vi "HAGAR_ECD.vi"() -> ()   [LabVIEW 2017]
uses:
  <vilib>/FPGAPlugInAG/cRIO-9035/niLvFpga_Close_cRIO-9035.vi
  <vilib>/rvi/errors/niLvFpgaAdjustHostInterfaceError.vi
  <vilib>/Utility/error.llb/Error Cluster From Error Code.vi
  GVZeitenZyklen_ECD.vi
  gvbooleschRT_ECD.vi
  GVHorstSP_ECD.vi
  GVMethodenwechsel_ECD.vi
  GVaktuelleTDMS_ECD.vi
  GVChroms_ECD.vi
  GVMetavariablen_ECD.vi
  GVMWHorst_ECD.vi
  GVVentilposition_ECD.vi
  GVHK1Hz_ECD.vi
  GVZwangs_ECD.vi
  GVZwangsMPV_ECD.vi
  GVTrapsMachs_ECD.vi
  GVECDs_ECD.vi
  GVAIs_ECD.vi
  GVHeizenLH_ECD.vi
  GVProbenvol_ECD.vi
  GVZwischenspeicher.vi
  <vilib>/rvi/interface/nirviCloseFPGA/nirviCloseFPGA.xnode
  FPGA Bitfiles/HAGAR-V_FPGATargetECD_FPGA-ProgrammECD_LbBtUh8SPQY.lvbitx
  FPGA_ECD/FPGA-Programm_ECD.vi
  <vilib>/rvi/interface/nirviReadWriteControl/nirviReadWriteControl.xnode
  <vilib>/rvi/interface/nirviMethod/nirviMethod.xnode
  <vilib>/NI_Real-Time Target Support.lvlib
  <vilib>/rvi/errors/niLvFpgaMergeErrorWithErrorCode.vi
  <vilib>/FPGAPlugInAG/cRIO-9035/niLvFpga_WriteFifo_cRIO-9035.vi
  NiFpgaLv.dll
panel:
  in  "Zyklus":enum16{"Mod0", "Mod1", "Mod2A", "Mod2B"}(ring)=enum."Mod1"
  in  "am Ende benutzen":bool
  in  "Methode speichern":bool
  out "ZyklusNummernGesamt":i32[](array[numeric])
  in  "veränderte Methode benutzen":bool
  in  "Methode verändern":bool
  out "ZyklusNummern":i32[](array[numeric])
  out "Big Ben, Methodenzeit, Zykluszeit0, Zykluszeit1, Zykluszeit2A, Zykluszeit2B":i32[](array[numeric])
  in  "global stop RT":bool
  in  "Methode":i32(ring) items=["Bedingsmethode", "Startmethode", "Meßmodus", "Shut-up-Methode", "Test", "HAG2 1/2", "Startmethode", "HAG2 1/2 Aufwärmen", "LicorDruckProfil1", "LicorDruckProfil2", "LicorDruckProfil0", "LicorDruckProfil3", "Kalibration-Meßmodus", "Kalibration-Meßmodus-II", "Kalibration-MesmodusIII", "Kalibration-Messmodus-IV", "Kalibration-ECD", "", "Kalibration-ECD-Blank"]
  in  "Registerkarte":T1(tab)
  out "SHOK?":bool[](array[boolean])
  out "schnelle Heizungen":string[](array[string])
  out "schnelle Heizungen":dbl[](array[numeric])
  out "HorstOK?":bool[](array[boolean])
  out "AIs3OK?":bool[](array[boolean])
  out "AIs1OK?":bool[](array[boolean])
  out "AIs1":dbl[](array[numeric])
  out "AIs1":string[](array[string])
  out "AIs2":string[](array[string])
  out "AIs3":string[](array[string])
  out "AIs2":dbl[](array[numeric])
  out "AIs3":dbl[](array[numeric])
  out "Metavariablen":string[](array[string])
  out "MVWerte":dbl[](array[numeric])
  out "MWHorst":dbl[](array[numeric])
  out "HorstRegler":string[](array[string])
  out "AIs2OK?":bool[](array[boolean])
  out "Ventilposition":i32=1 min=1 max=6 step=1
  out "MVOK?":bool[](array[boolean])
  out "CPU Total (%)":dbl
  in  "MVFixwert":dbl[](array[numeric])
  in  "MVFix?":bool[](array[boolean])
  in  "LH-Gruppe":bool[](array[boolean])=[FALSE, FALSE, FALSE, FALSE, FALSE, FALSE, FALSE, FALSE, FALSE, FALSE, FALSE, FALSE]
  out "LangsameHeizungen":string[](array[string])
  out "Housekeeping1":cluster{dbl[], dbl[]}(graph)
  in  "Zeitachse1":i32(ring)=1 items=["Zykluszeit [s] Mod0", "Zykluszeit [s] Mod1", "Zykluszeit [s] Mod2A", "Zykluszeit [s] Mod2B"]
  in  "dargestellte Größe 1":i32(ring)=1 items=["T1-Spare1", "T1-Spare2", "T1-StirlingKühlkopf [°C]", "T1-PreCol1 [°C]", "T1-PreCol2 [°C]", "T1-MainCol1a [°C]", "T1-MainCol1b [°C]", "T1-MainCol2a [°C]", "T1-MainCol2b [°C]", "T1-BronkhorstUntena [°C]", "T1-BronkhorstUntenb [°C]", "T1-BronkhorstObena [°C]", "T1-BronkhorstObenb [°C]", "T1-2Pos1B [°C]", "T1-Spare9", "T1-2Pos1A [°C]", "T1-Spare10", "T1-TurboPump [°C]", "T1-StirlingPlatine [°C]", "T1-Spare5", "T1-Spare6", "T1-Spare7", "T1-Inlet [°C]", "F1-MFM-Spare", "F1-MFM0D [mL]", "P1-HeliumHP [bara]", "P1-HeliumLP [bara]", "P1-PumpVordruck [mbara]", "TurboSpeed", "I1-MS-AC [A]", "I1-Trap1 [A]", "I1-Trap2 [A]", "T2-ECD1a", "T2-ECD1b", "T2-ECD2a", "T2-ECD2b", "T2-Col1a", "T2-Col1b", "T2-Col2a", "T2-Col2b", "T2-Spare1", "T2-Spare2", "T2-Spare3", "T2-Spare4", "T2-Spare5", "T2-Spare6", "T2-Spare7", "F2-MFM2A", "F2-MFM2B", "F2-MFM2C", "P2-N2O_HP", "P2-N2O_LP", "P2-CO2_HP", "P2-CO2_LP", "AI-Spare1", "FL-MFM1000mL", "AI-Spare3", "AI-Spare4", "StirlingAlarm", "StirlingEmerg.", "AI-Spare7", "AI-Spare8", "AI-Spare9", "FL-MFM30mL", "T0-DC/DC5", "I0-24V_M0", "I0-48V_M1", "I0-24V_M1", "I0-28V_M2", "T0-Spare3", "T0-Spare2", "T0-Spare4", "T0-DC/DC7", "I0-20V_Laptop", "I0-28V_M1", "I0-24V_M2", "I0-12V_Licor", "T0-Spare1", "T0-Drier", "T0-Spare5", "F0-MFM0A [L]", "TL-Licor_a", "P0-Span-HP", "P0-spare1", "P0-Stickstoff-LP", "P0-Helium-LP", "P0-Cal-HP", "P0-P9Tavco[bar]", "F0-MFM0B [L]", "TL-Licor_b", "P0-Span-LP", "P0-spare2", "P0-Stickstoff-HP", "P0-Helium-HP", "P0-Cal-LP", "F0-MFM3", "Trap1 [°C]", "Trap2 [°C]", "PreCol1 [°C]", "PreCol2 [°C]", "MainCol1 [°C]", "MainCol2 [°C]", "PrC0 [bara]", "PrC0-Licor [bara]", "PrC1-Säule1 [bara]", "PrC1-Säule2 [bara]", "MFC1-Sample [ml/min]", "PrC1-BackFlush1 [bara]", "PrC1-BackFlush2 [bara]", "MFC1-Reaktant [l/min]", "MFC2A[ml/min]", "MFC2B[ml/min]", "MFC2C[ul/min]", "PrC2A[bara]", "MFC2D[ml/min]", "MFC2E[ml/min]", "PrC2B[bara]"]
  out "Housekeeping2":cluster{dbl[], dbl[]}(graph)
  in  "Zeitachse2":i32(ring)=1 items=["Zykluszeit [s] Mod0", "Zykluszeit [s] Mod1", "Zykluszeit [s] Mod2A", "Zykluszeit [s] Mod2B"]
  in  "dargestellte Größe 2":i32(ring)=1 items=["T1-Spare1", "T1-Spare2", "T1-StirlingKühlkopf [°C]", "T1-PreCol1 [°C]", "T1-PreCol2 [°C]", "T1-MainCol1a [°C]", "T1-MainCol1b [°C]", "T1-MainCol2a [°C]", "T1-MainCol2b [°C]", "T1-BronkhorstUntena [°C]", "T1-BronkhorstUntenb [°C]", "T1-BronkhorstObena [°C]", "T1-BronkhorstObenb [°C]", "T1-2Pos1B [°C]", "T1-Spare9", "T1-2Pos1A [°C]", "T1-Spare10", "T1-TurboPump [°C]", "T1-StirlingPlatine [°C]", "T1-Spare5", "T1-Spare6", "T1-Spare7", "T1-Inlet [°C]", "F1-MFM-Spare", "F1-MFM0D [mL]", "P1-HeliumHP [bara]", "P1-HeliumLP [bara]", "P1-PumpVordruck [mbara]", "TurboSpeed", "I1-MS-AC [A]", "I1-Trap1 [A]", "I1-Trap2 [A]", "T2-ECD1a", "T2-ECD1b", "T2-ECD2a", "T2-ECD2b", "T2-Col1a", "T2-Col1b", "T2-Col2a", "T2-Col2b", "T2-Spare1", "T2-Spare2", "T2-Spare3", "T2-Spare4", "T2-Spare5", "T2-Spare6", "T2-Spare7", "F2-MFM2A", "F2-MFM2B", "F2-MFM2C", "P2-N2O_HP", "P2-N2O_LP", "P2-CO2_HP", "P2-CO2_LP", "AI-Spare1", "FL-MFM1000mL", "AI-Spare3", "AI-Spare4", "StirlingAlarm", "StirlingEmerg.", "AI-Spare7", "AI-Spare8", "AI-Spare9", "FL-MFM30mL", "T0-DC/DC5", "I0-24V_M0", "I0-48V_M1", "I0-24V_M1", "I0-28V_M2", "T0-Spare3", "T0-Spare2", "T0-Spare4", "T0-DC/DC7", "I0-20V_Laptop", "I0-28V_M1", "I0-24V_M2", "I0-12V_Licor", "T0-Spare1", "T0-Drier", "T0-Spare5", "F0-MFM0A [L]", "TL-Licor_a", "P0-Span-HP", "P0-spare1", "P0-Stickstoff-LP", "P0-Helium-LP", "P0-Cal-HP", "P0-P9Tavco[bar]", "F0-MFM0B [L]", "TL-Licor_b", "P0-Span-LP", "P0-spare2", "P0-Stickstoff-HP", "P0-Helium-HP", "P0-Cal-LP", "F0-MFM3", "Trap1 [°C]", "Trap2 [°C]", "PreCol1 [°C]", "PreCol2 [°C]", "MainCol1 [°C]", "MainCol2 [°C]", "PrC0 [bara]", "PrC0-Licor [bara]", "PrC1-Säule1 [bara]", "PrC1-Säule2 [bara]", "MFC1-Sample [ml/min]", "PrC1-BackFlush1 [bara]", "PrC1-BackFlush2 [bara]", "MFC1-Reaktant [l/min]", "MFC2A[ml/min]", "MFC2B[ml/min]", "MFC2C[ul/min]", "PrC2A[bara]", "MFC2D[ml/min]", "MFC2E[ml/min]", "PrC2B[bara]"]
  out "Detektor 2":cluster{dbl[], dbl[]}[](graph)
  in  "Detektor":i32(ring) items=["ECD1", "ECD2"]
  in  "HK1YMin":dbl
  in  "HK1YMax":dbl=100.0
  in  "HK2YMin":dbl
  in  "HK2YMax":dbl=100.0
  in  "DetYMin":dbl
  in  "DetYMax":dbl=100.0
  in  "NeuerRefstrom":bool
  in  "RefStromECD1":i16=800 min=0 max=2500 step=1
  in  "RefStromECD2":i16=2100 min=0 max=2500 step=1
  out "schnelleAnzeige":cluster{dbl[], dbl[]}(graph)
  in  "TafelWischen!":bool
  in  "dargestellte Größe 3":i32(ring)=1 items=["Trap1 [°C]", "Trap2 [°C]", "PreCol1 [°C]", "PreCol2 [°C]", "MainCol1 [°C]", "MainCol2 [°C]", "PrC0 [bara]", "PrC0-Licor [bara]", "PrC1-Säule1 [bara]", "PrC1-Säule2 [bara]", "MFC1-Sample [ml/min]", "PrC1-BackFlush1 [bara]", "PrC1-BackFlush2 [bara]", "MFC1-Reaktant [l/min]", "MFC2A[ml/min]", "MFC2B[ml/min]", "MFC2C[ul/min]", "PrC2A[bara]", "MFC2D[ml/min]", "MFC2E[ml/min]", "PrC2B[bara]"]
  in  "An/Aus":bool
  out "TDMSwriteECD":errorcluster
  out "AIsFIFOread":errorcluster
  out "MWTrapsMachs":errorcluster
  out "TDMSwriteHK":errorcluster
  out "TDMScloseHK":errorcluster
  out "TDMSopenHK":errorcluster
  out "TDMScloseECD2":errorcluster
  out "TDMSopenECD2":errorcluster
  out "TDMScloseECD1":errorcluster
  out "TDMSopenECD1":errorcluster
  out "FIFOwriteRS485":errorcluster
  out "SerielleKomm.":errorcluster
  out "LH":errorcluster
  out "Zyklus":errorcluster
  out "ECD1dataBackup":errorcluster
  out "ECD2dataBackup":errorcluster
  # "Zyklen:   ===>>"
  # "MS"
  # "ECD1"
  # "ECD2"
  # "Zykluszeiten:   ===>>"
  # "MS"
  # "ECD1"
  # "ECD2"
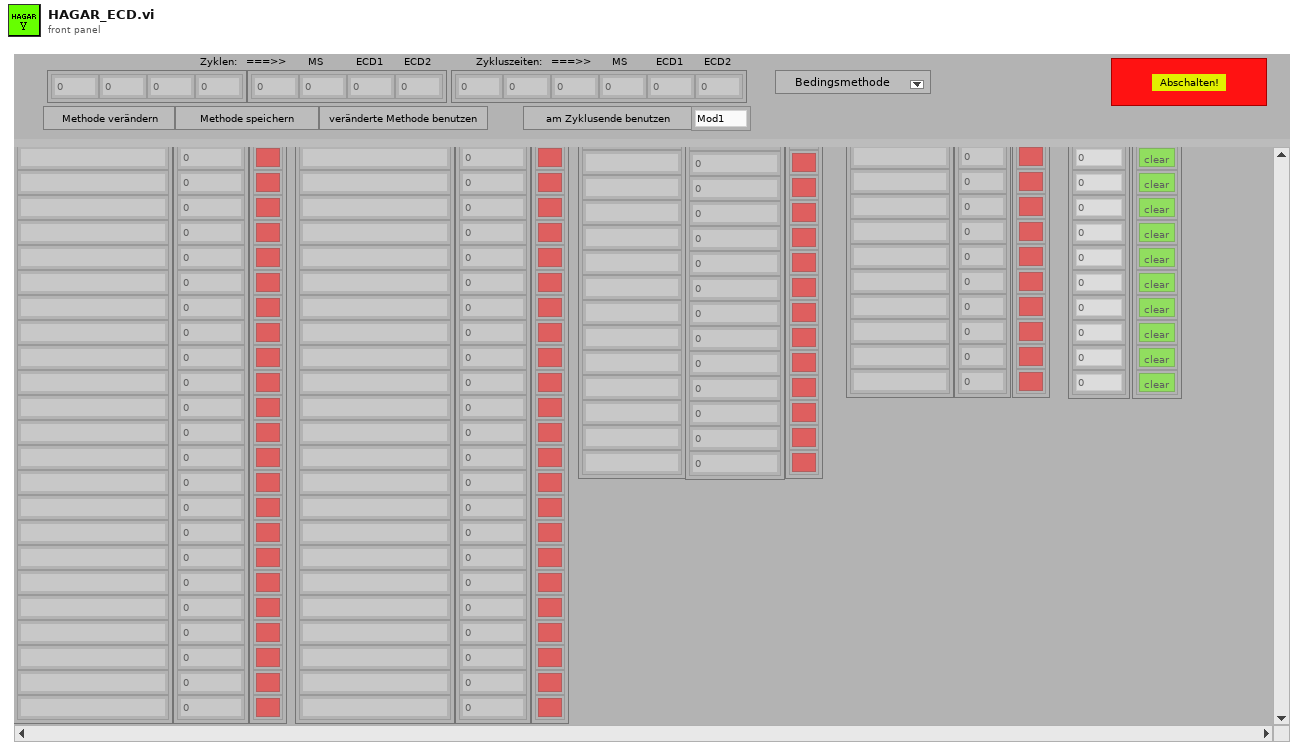
[diagram p1: front panel]
types:
  T1 = enum32{"Tabellen", "Heizungen gruppieren", "Bilder", "schnelle Bilder", "LICÖRchen", "Ups! Fehler"}
  T2 = cluster{"Zykluslängen [s]":dbl[], "ZeitpktDIOsMod0":dbl[], "ZeitpktDIOsMod1":dbl[], "ZeitpktDIOsMod2A":dbl[], "ZeitpktDIOsMod2B":dbl[], "DIOsSPMod0":bool[][], "DIOsSPMod1":bool[][], "DIOsSPMod2A":bool[][], "DIOsSPMod2B":bool[][], "Mod0HorstZeitpkt":dbl[], "Mod1HorstZeitpkt":dbl[], "Mod2AHorstZeitpkt":dbl[], "Mod2BHorstZeitpkt":dbl[], "HorstSPMod0":dbl[][], "HorstSPMod1":dbl[][], "HorstSPMod2A":dbl[][], "HorstSPMod2B":dbl[][], "LHSetpoints":dbl[], "LHHeizen?":bool[], "ZPktFPGABoolesch":dbl[], "FPGABoolesch":bool[][], "ZeitpktFPGAPID":dbl[], "FPGAPID":cluster{"d0":fxp<+/-,18,18>, "d1":fxp<+/-,21,21>}[][], "ZeitpktFPGAFixp":dbl[], dbl[][], "t_PreMach1":dbl[], "T_PreMach1":dbl[], "t_PreMach2":dbl[], "T_PreMach2":dbl[], "PIDs für \"träge\" Heizungen":cluster{"proportional gain (Kc)":dbl, "integral time (Ti, min)":dbl, "derivative time (Td, min)":dbl}[], "Zwangsbedingungen":dbl[][], "Dateien fürs MS schicken?":bool, "ZeitpunkteMPV":dbl[], "SPMPV":i32[], "ZeitpktMS-1":dbl, "ZeitpktMS-2":dbl, "Int.Start1":dbl, "Int.Stop1":dbl, "Int.Start2":dbl, "Int.Stop2":dbl, "Methodenname":string, "t_MainMach1":dbl[], "T_MainMach1":dbl[], "t_MainMach2":dbl[], "T_MainMach2":dbl[]}[]
  T3 = cluster{"DIOsMod0Nr":i32[], "DIOsMod1Nr":i32[], "DIOsMod2ANr":i32[], "DIOsMod2BNr":i32[], "AIsLH":i32[], "AnzahlRegler/Modul":i32[], "Regler für den Probenfluß":i32, "SPvorgebenMod0":string[], "SPvorgebenMod1":string[], "SPvorgebenMod2A":string[], "SPvorgebenMod2B":string[], "MWAntwortMod0":string[], "MWAntwortMod1":string[], "MWAntwortMod2A":string[], "MWAntwortMod2B":string[], "FaktorMod0":dbl[], "FaktorMod1":dbl[], "FaktorMod2A":dbl[], "FaktorMod2B":dbl[], "MWabfragenMod0":string[], "MWabfragenMod1":string[], "MWabfragenMod2A":string[], "MWabfragenMod2B":string[], "Modul1/AI koeff":dbl[][], "Modul2/AI koeff":dbl[][], "Modul3/AI koeff":dbl[][], "Traps/MachsKoeff T(R)":dbl[][], "Modul1/AIsNamen":string[], "Modul2/AIsNamen":string[], "Modul3/AIsNamen":string[], "DIOsMod0Name":string[], "DIOsMod1Name":string[], "DIOsMod2AName":string[], "DIOsMod2BName":string[], "ReglerNameMod0":string[], "ReglerNameMod1":string[], "ReglerNameMod2A":string[], "ReglerNameMod2B":string[], "Startmethode":i32, "Dateiordner Housekeeping":path, "Dateiname Housekeeping":string, "DateiordnerECD1":path, "DateinameECD1":string, "DateiordnerECD2":path, "DateinameECD2":string, "LangsameHeizungen":string[], "ModuleLH":i32[], "Metavariablen":string[], "Modul1/AI sicherer Bereich":dbl[][], "Modul2/AI sicherer Bereich":dbl[][], "Modul3/AI sicherer Bereich":dbl[][], "Traps/Machs sicherer Bereich":dbl[][], "ReglerMod0 sicherer Bereich":dbl[][], "ReglerMod1 sicherer Bereich":dbl[][], "ReglerMod2A sicherer Bereich":dbl[][], "ReglerMod2B sicherer Bereich":dbl[][], "Metavariablen grüner Bereich":dbl[][], "Traps/MachsKoeff R(U)":dbl[][], "LHGruppe":bool[]}
  T4 = enum16{"open", "replace", "create", "open or create", "replace or create", "replace or create with confirmation"}
  T5 = cluster{"Zyklus1":i32, "Zeitachse1":i32, "dargestellte Größe 1":i32, "Zyklus2":i32, "Zeitachse2":i32, "dargestellte Größe 2":i32}
  T6 = cluster{"DIOsMod0Name":string[], "DIOsMod1Name":string[], "DIOsMod2AName":string[], "DIOsMod2BName":string[], "ReglerNameMod0":string[], "ReglerNameMod1":string[], "ReglerNameMod2A":string[], "ReglerNameMod2B":string[], "LangsameHeizungen":string[]}
  T7 = cluster{"Zykluslängen [s]":dbl[], "ZeitpktDIOsMod0":dbl[], "ZeitpktDIOsMod1":dbl[], "ZeitpktDIOsMod2A":dbl[], "ZeitpktDIOsMod2B":dbl[], "DIOsSPMod0":bool[][], "DIOsSPMod1":bool[][], "DIOsSPMod2A":bool[][], "DIOsSPMod2B":bool[][], "Mod0HorstZeitpkt":dbl[], "Mod1HorstZeitpkt":dbl[], "Mod2AHorstZeitpkt":dbl[], "Mod2BHorstZeitpkt":dbl[], "HorstSPMod0":dbl[][], "HorstSPMod1":dbl[][], "HorstSPMod2A":dbl[][], "HorstSPMod2B":dbl[][], "LHSetpoints":dbl[], "LHHeizen?":bool[], "ZPktFPGABoolesch":dbl[], "FPGABoolesch":bool[][], "ZeitpktFPGAPID":dbl[], "FPGAPID":cluster{"d0":fxp<+/-,18,18>, "d1":fxp<+/-,21,21>}[][], "ZeitpktFPGAFixp":dbl[], dbl[][], "t_PreMach1":dbl[], "T_PreMach1":dbl[], "t_PreMach2":dbl[], "T_PreMach2":dbl[], "PIDs für \"träge\" Heizungen":cluster{"proportional gain (Kc)":dbl, "integral time (Ti, min)":dbl, "derivative time (Td, min)":dbl}[], "Zwangsbedingungen":dbl[][], "Dateien fürs MS schicken?":bool, "ZeitpunkteMPV":dbl[], "SPMPV":i32[], "ZeitpktMS-1":dbl, "ZeitpktMS-2":dbl, "Int.Start1":dbl, "Int.Stop1":dbl, "Int.Start2":dbl, "Int.Stop2":dbl, "Methodenname":string, "t_MainMach1":dbl[], "T_MainMach1":dbl[], "t_MainMach2":dbl[], "T_MainMach2":dbl[]}
  T8 = cluster{"Modul1/AI sicherer Bereich":dbl[][], "Modul2/AI sicherer Bereich":dbl[][], "Modul3/AI sicherer Bereich":dbl[][], "Traps/Machs sicherer Bereich":dbl[][], dbl[][], "Metavariablen grüner Bereich":dbl[][]}
  T9 = cluster{"created path":path, "created path":path}
  T10 = cluster{"created path":path, "created path":path, "created path":path, "Dateiname Housekeeping":string, "DateinameECD1":string, "DateinameECD2":string, "tdms0":refnum<k34>, "tdms1":refnum<k34>, "tdms0":refnum<k34>, "tdms1":refnum<k34>, "tdms0":refnum<k34>, "tdms1":refnum<k34>}
  T11 = cluster{"d0":fxp<+/-,18,18>, "d1":fxp<+/-,21,21>}[][]
  T12 = cluster{"proportional gain (Kc)":dbl, "integral time (Ti, min)":dbl, "derivative time (Td, min)":dbl}[]
  T13 = cluster{cluster{"ZeitpktDIOsMod2B":dbl[]}[], cluster{"DIOsSPMod2B":bool[][]}[], cluster{"Mod2BHorstZeitpkt":dbl[]}[], cluster{"HorstSPMod2B":dbl[][]}[], "LHHeizen?":bool[], "ZPktFPGABoolesch":dbl[], "FPGABoolesch":bool[][], "ZeitpktFPGAPID":dbl[], "FPGAPID":cluster{"d0":fxp<+/-,18,18>, "d1":fxp<+/-,21,21>}[][], "ZeitpktFPGAFixp":dbl[], dbl[][], "t_PreMach1":dbl[], "T_PreMach1":dbl[], "t_PreMach2":dbl[], "T_PreMach2":dbl[], "ZeitpunkteMPV":dbl[], "SPMPV":i32[], "t_MainMach1":dbl[], "T_MainMach1":dbl[], "t_MainMach2":dbl[], "T_MainMach2":dbl[]}
  T14 = cluster{"Zykluslängen [s]":dbl[], "ZeitpktDIOsMod0":dbl[], "ZeitpktDIOsMod1":dbl[], "ZeitpktDIOsMod2A":dbl[], "ZeitpktDIOsMod2B":dbl[], "DIOsSPMod0":bool[][], "DIOsSPMod1":bool[][], "DIOsSPMod2A":bool[][], "DIOsSPMod2B":bool[][], "Mod0HorstZeitpkt":dbl[], "Mod1HorstZeitpkt":dbl[], "Mod2AHorstZeitpkt":dbl[], "Mod2BHorstZeitpkt":dbl[], "HorstSPMod0":dbl[][], "HorstSPMod1":dbl[][], "HorstSPMod2A":dbl[][], "HorstSPMod2B":dbl[][], "LangsameHeizungenSP":dbl[], "LHHeizen?":bool[], "ZPktFPGABoolesch":dbl[], "FPGABoolesch":bool[][], "ZeitpktFPGAPID":dbl[], "FPGAPID":cluster{"d0":fxp<+/-,18,18>, "d1":fxp<+/-,21,21>}[][], "ZeitpktFPGAFixp":dbl[], "FPGAFixp":dbl[][], "t_PreMach1":dbl[], "T_PreMach1":dbl[], "t_PreMach2":dbl[], "T_PreMach2":dbl[], "PIDs für \"träge\" Heizungen":cluster{"proportional gain (Kc)":dbl, "integral time (Ti, min)":dbl, "derivative time (Td, min)":dbl}[], "Zwangsbedingungen":dbl[][], "MS-Daten?":bool, "ZeitpunkteMPV":dbl[], "SetpointMPV":i32[], "ZeitpktMS-1":dbl, "ZeitpktMS-2":dbl, "Int.Start1":dbl, "Int.Stop1":dbl, "Int.Start2":dbl, "Int.Stop2":dbl, "Methodenname":string, "t_MainMach1":dbl[], "T_MainMach1":dbl[], "t_MainMach2":dbl[], "T_MainMach2":dbl[]}
  T15 = cluster{"ZyklusNummern":i32[], "ZeilennummernDIOs":i32[], "ZwangsDIO?":cluster{bool[]}[], "ZeilennummernHorst":i32[], "ZwangsHorst?":cluster{bool[]}[], "ZeileFPGABoolesch":i32, "ZwangsFPGABoolesch?":bool[], "ZeileFPGAPID":i32, "ZeileFPGAFixp":i32, "ZeilePreMach1":i32, "ZeilePreMach2":i32, "ZeilennummerMPV":i32, "ZeileMainMach1":i32, "ZeileMainMach2":i32, "ZwangsMPV?":bool}
  T16 = typedef "NI_Real-Time Target Support.lvlib/RT CPU Load.ctl" = cluster{"Total (%)":dbl, "Time Critical (%)":dbl, "Timed Structures (%)":dbl, "High (%)":dbl, "Above Normal (%)":dbl, "Normal (%)":dbl, "Background (%)":dbl, "Idle (%)":dbl, "ISR (%)":dbl}
  T17 = cluster{"ZyklusNummern":i32[], i32[], "ZwangsDIO?":cluster{bool[]}[], i32[], "ZwangsHorst?":cluster{bool[]}[], i32, "ZwangsFPGABoolesch?":bool[], i32, i32, "ZeileMach":i32, "ZeileMach":i32, i32, "ZeileMach":i32, "ZeileMach":i32, "ZwangsMPV?":bool}
  T18 = cluster{string[], string[], string[], dbl[], dbl[], dbl[]}
  T19 = cluster{"Befehle1":string[], "Befehle2":string[], "Befehle3":string[]}
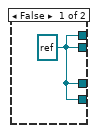
[diagram p2: hidden frame]
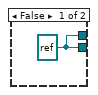
[diagram p3: hidden frame]
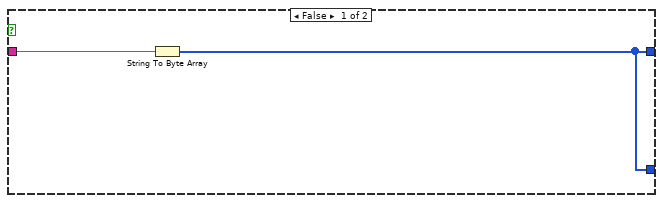
[diagram p6: hidden frame]
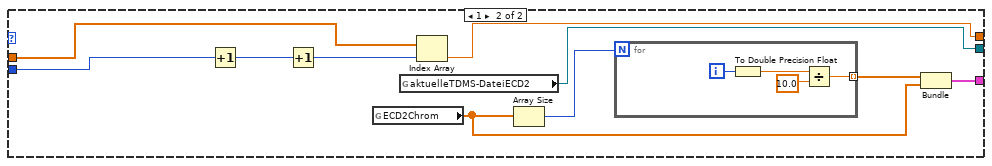
[diagram p16: hidden frame]
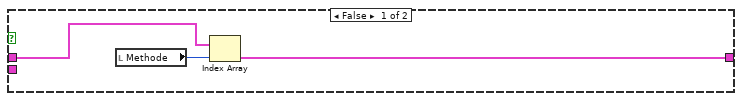
[diagram p17: hidden frame]
diagram:
  w2 = path "c:/methoden.pery" ("Datei (Dialog verwenden)")
  w3 = path "c:/einstellungen.pery" ("Datei (Dialog verwenden)")
  n1 = Open/Create/Replace File(file path (use dialog)=w3, operation (0:open)=T4."open" ("Operation (0:Öffnen)")) -> (refnum out=w15:refnum<file>)  [unwired: 4 in, 2 out]
  n2 = Open/Create/Replace File(file path (use dialog)=w2, operation (0:open)=T4."open" ("Operation (0:Öffnen)")) -> (refnum out=w11:refnum<file>)  [unwired: 4 in, 2 out]
  n3 = Read from Binary File(5:T3 {"DIOsMod0Nr"=[], "DIOsMod1Nr"=[], "DIOsMod2ANr"=[], "DIOsMod2BNr"=[], "AIsLH"=[], "AnzahlRegler/Modul"=[], "Regler für den Probenfluß"=0, "SPvorgebenMod0"=[], "SPvorgebenMod1"=[], "SPvorgebenMod2A"=[], "SPvorgebenMod2B"=[], "MWAntwortMod0"=[], "MWAntwortMod1"=[], "MWAntwortMod2A"=[], "MWAntwortMod2B"=[], "FaktorMod0"=[], "FaktorMod1"=[], "FaktorMod2A"=[], "FaktorMod2B"=[], "MWabfragenMod0"=[], "MWabfragenMod1"=[], "MWabfragenMod2A"=[], "MWabfragenMod2B"=[], "Modul1/AI koeff"=[], "Modul2/AI koeff"=[], "Modul3/AI koeff"=[], "Traps/MachsKoeff T(R)"=[], "Modul1/AIsNamen"=[], "Modul2/AIsNamen"=[], "Modul3/AIsNamen"=[], "DIOsMod0Name"=[], "DIOsMod1Name"=[], "DIOsMod2AName"=[], "DIOsMod2BName"=[], "ReglerNameMod0"=[], "ReglerNameMod1"=[], "ReglerNameMod2A"=[], "ReglerNameMod2B"=[], "Startmethode"=0, "Dateiordner Housekeeping"=path "", "Dateiname Housekeeping"="", "DateiordnerECD1"=path "", "DateinameECD1"="", "DateiordnerECD2"=path "", "DateinameECD2"="", "LangsameHeizungen"=[], "ModuleLH"=[], "Metavariablen"=[], "Modul1/AI sicherer Bereich"=[], "Modul2/AI sicherer Bereich"=[], "Modul3/AI sicherer Bereich"=[], "Traps/Machs sicherer Bereich"=[], "ReglerMod0 sicherer Bereich"=[], "ReglerMod1 sicherer Bereich"=[], "ReglerMod2A sicherer Bereich"=[], "ReglerMod2B sicherer Bereich"=[], "Metavariablen grüner Bereich"=[], "Traps/MachsKoeff R(U)"=[], "LHGruppe"=[]} ("output cluster"), 11:w15) -> (2:w13:T3, 3:w14:refnum<file>)  [unwired: 4 in, 2 out]
  n4 = Read from Binary File(5:T2 [], 11:w11) -> (2:w9:T2, 3:w10:refnum<file>)  [unwired: 4 in, 2 out]
  n5 = Close File(refnum=w14) -> ()  [unwired: 1 in, 2 out]
  n6 = Close File(refnum=w10) -> ()  [unwired: 1 in, 2 out]
  n7 = flat-sequence {
    tunnel: [w86] -> w42
    tunnel: [w146] -> w41
    tunnel: [w89] -> w39
    tunnel: [w279] -> w38
    tunnel: [w281] -> w37
    tunnel: [w273] -> w36
    tunnel: [w280] -> w35
    tunnel: [w203] -> w34
    tunnel: [w272] -> w33
    tunnel: [w271] -> w32
    tunnel: [w265] -> w31
    tunnel: [w206] -> w30
    tunnel: [w180] -> w29
    tunnel: [w278] -> w28
    tunnel: [w270] -> w27
    tunnel: [w269] -> w26
    tunnel: [w261] -> w25
    tunnel: [w260] -> w24
    tunnel: [w259] -> w23
    tunnel: [w258] -> w22
    tunnel: [w257] -> w21
    tunnel: [w256] -> w20
    tunnel: [w253] -> w19
    tunnel: [w235] -> w18
    tunnel: w13 -> [w128]
    tunnel: [w234] -> w17
    tunnel: w9 -> [w147]
    tunnel: [w146] -> w8
    tunnel: [w128] -> w7
    tunnel: [w97] -> w6
    tunnel: w3 -> [w83]
    tunnel: w2 -> [w79]
    tunnel: [w60] -> w1
    tunnel: w42 -> [w347]
    tunnel: w41 -> [w420]
    tunnel: [w347] -> w40
    tunnel: w39 -> [_]
    tunnel: w38 -> [w378]
    tunnel: w37 -> [w377]
    tunnel: w36 -> [w379]
    tunnel: w35 -> [w376]
    tunnel: w34 -> [w351]
    tunnel: w33 -> [w346]
    tunnel: w32 -> [w343]
    tunnel: w31 -> [w340]
    tunnel: w30 -> [w341]
    tunnel: w29 -> [w344]
    tunnel: w28 -> [w418]
    tunnel: w27 -> [w349]
    tunnel: w26 -> [w419]
    tunnel: w25 -> [w322]
    tunnel: w24 -> [w321]
    tunnel: w23 -> [w320]
    tunnel: w22 -> [w416]
    tunnel: w21 -> [w415]
    tunnel: w20 -> [w414]
    tunnel: w19 -> [w368]
    tunnel: w18 -> [w350]
    tunnel: w17 -> [w339]
    tunnel: w9 -> [w338]
    tunnel: w8 -> [w336]
    tunnel: w7 -> [_]
    tunnel: w6 -> [w315]
    tunnel: w1 -> [w314]
    tunnel: w40 -> [w1212]
    frame #0 {
      w43 = string[] ["x", "x", "x", "x"] ("write")
      w56 = "config" ("string")
      w78 = string[] ["Trap1 [°C]", "Trap2 [°C]", "PreCol1 [°C]", "PreCol2 [°C]", "MainCol1 [°C]", "MainCol2 [°C]"]
      w148 = TRUE
      w162 = 0.0 ("Probenvol.1")
      w169 = dbl[] [-1.0] ("ECD1MW")
      w170 = FALSE ("ECD1Empfangen?")
      w276 = string[] ["Big Ben [s]", "Methodenzeit [s]", "Zykluszeit [s] Mod0", "Zykluszeit [s] Mod1", "Zykluszeit [s] Mod2A", "Zykluszeit [s] Mod2B"]
      w266 = FALSE ("Undefinierte Werte möglich")
      w267 = FALSE ("global stop RT")
      n8 = for {
        tunnel: [w309] -> w274 mode=indexing
        tunnel: w147 -> [w310] mode=indexing
        n9 = Unbundle(w310) -> ("Methodenname"=w309:string)  [unwired: 44 out]
      }
      n10 = Unbundle(w128) -> ("DIOsMod0Nr"=w190:i32[], "DIOsMod1Nr"=w189:i32[], "DIOsMod2ANr"=w188:i32[], "DIOsMod2BNr"=w187:i32[], "AIsLH"=w177:i32[], "AnzahlRegler/Modul"=w180:i32[], "Regler für den Probenfluß"=w234:i32, "SPvorgebenMod0"=w233:string[], "SPvorgebenMod1"=w232:string[], "SPvorgebenMod2A"=w231:string[], "SPvorgebenMod2B"=w230:string[], "MWAntwortMod0"=w229:string[], "MWAntwortMod1"=w228:string[], "MWAntwortMod2A"=w227:string[], "MWAntwortMod2B"=w226:string[], "FaktorMod0"=w225:dbl[], "FaktorMod1"=w224:dbl[], "FaktorMod2A"=w223:dbl[], "FaktorMod2B"=w222:dbl[], "MWabfragenMod0"=w221:string[], "MWabfragenMod1"=w220:string[], "MWabfragenMod2A"=w219:string[], "MWabfragenMod2B"=w218:string[], "Modul1/AI koeff"=w217:dbl[][], "Modul2/AI koeff"=w216:dbl[][], "Modul3/AI koeff"=w215:dbl[][], "Traps/MachsKoeff T(R)"=w214:dbl[][], "Modul1/AIsNamen"=w213:string[], "Modul2/AIsNamen"=w212:string[], "Modul3/AIsNamen"=w211:string[], "DIOsMod0Name"=w126:string[], "DIOsMod1Name"=w127:string[], "DIOsMod2AName"=w125:string[], "DIOsMod2BName"=w124:string[], "ReglerNameMod0"=w139:string[], "ReglerNameMod1"=w138:string[], "ReglerNameMod2A"=w137:string[], "ReglerNameMod2B"=w136:string[], "Startmethode"=w146:i32, "Dateiordner Housekeeping"=w65:path, "Dateiname Housekeeping"=w210:string, "DateiordnerECD1"=w70:path, "DateinameECD1"=w209:string, "DateiordnerECD2"=w62:path, "DateinameECD2"=w208:string, "LangsameHeizungen"=w207:string[], "ModuleLH"=w202:i32[], "Metavariablen"=w141:string[], "Modul1/AI sicherer Bereich"=w101:dbl[][], "Modul2/AI sicherer Bereich"=w100:dbl[][], "Modul3/AI sicherer Bereich"=w99:dbl[][], "Traps/Machs sicherer Bereich"=w98:dbl[][], "ReglerMod0 sicherer Bereich"=w96:dbl[][], "ReglerMod1 sicherer Bereich"=w95:dbl[][], "ReglerMod2A sicherer Bereich"=w94:dbl[][], "ReglerMod2B sicherer Bereich"=w93:dbl[][], "Metavariablen grüner Bereich"=w91:dbl[][], "LHGruppe"=w85:bool[])  [unwired: 1 out]
      "Metavariablen" <- w141
      "LangsameHeizungen" <- w207
      n11 = Initialize Array(0, 4 ("Dimension")) -> (w163:i32[])
      n12 = Initialize Array(0.0 ("Element"), 6 ("Dimension")) -> (w166:dbl[])
      n13 = global write "GVMethodenwechsel_ECD.vi" "Methodenwechsel?"(FALSE ("Methodenwechsel?")) -> ()
      n14 = local write "NeuerRefstrom"(FALSE ("NeuerRefstrom")) -> ()
      n15 = property on="dargestellte Größe 2" class="Ring (strikt)"("AllowUndefVals"=w266) -> ()  [unwired: 2 in, 2 out]
      n16 = property on="Zeitachse2" class="Ring (strikt)"("AllowUndefVals"=w266) -> ()  [unwired: 2 in, 2 out]
      n17 = property on="Zeitachse1" class="Ring (strikt)"("AllowUndefVals"=w266) -> ()  [unwired: 2 in, 2 out]
      n18 = property on="dargestellte Größe 1" class="Ring (strikt)"("AllowUndefVals"=w266) -> ()  [unwired: 2 in, 2 out]
      n19 = property on="Methode" class="Ring (strikt)"("AllowUndefVals"=w266) -> ()  [unwired: 2 in, 2 out]
      n20 = global write "GVProbenvol_ECD.vi" "Probenvol.1"(w162) -> ()
      n21 = global write "GVProbenvol_ECD.vi" "Probenvol.2"(w162) -> ()
      n22 = global write "GVECDs_ECD.vi" "ECD1MW"(w169) -> ()
      n23 = global write "GVECDs_ECD.vi" "ECD2MW"(w169) -> ()
      n24 = global write "GVECDs_ECD.vi" "ECD1Empfangen?"(w170) -> ()
      n25 = global write "GVECDs_ECD.vi" "ECD2Empfangen?"(w170) -> ()
      n26 = local write "global stop RT"(w267) -> ()
      n27 = global write "gvbooleschRT_ECD.vi" "global stop RT"(w267) -> ()
      n28 = global write "GVZeitenZyklen_ECD.vi" "ZyklusNummern"(w163) -> ()
      n29 = global write "GVZeitenZyklen_ECD.vi" "ZyklusNummernGesamt"(w163) -> ()
      n30 = global write "GVZeitenZyklen_ECD.vi" "Big Ben, Methodenzeit, Zykluszeit0, Zykluszeit1, Zykluszeit2A, Zykluszeit2B"(w166) -> ()
      n31 = property on="Methode" class="Ring (strikt)"("Value"=w146) -> ()  [unwired: 2 in, 2 out]
      n32 = Initialize Array(-1.0 ("Element"), 6 ("Dimension")) -> (w173:dbl[])
      n33 = Initialize Array(FALSE, 10 ("Dimension")) -> (w181:bool[])
      n34 = Initialize Array(-1.0 ("Element"), 96 ("Dimension")) -> (w174:dbl[])
      n35 = local write "LH-Gruppe"(w85) -> ()
      n36 = Strip Path(path=w65) -> (stripped path=w66:path)  [unwired: 1 out]
      n37 = Strip Path(path=w70) -> (stripped path=w67:path, name=w69:string)
      n38 = global write "GVZwangs_ECD.vi" "ZwangsFPGABoolesch!"(w181) -> ()
      n39 = global write "GVZwangs_ECD.vi" "ZwangsFPGABoolesch?"(w181) -> ()
      n40 = global write "GVTrapsMachs_ECD.vi" "Traps/Machs"(w173) -> ()
      n41 = global write "GVAIs_ECD.vi" "AIs"(w174) -> ()
      n42 = for {
        tunnel: w180 -> [w287] mode=indexing
        tunnel: [w284] -> w179 mode=indexing
        tunnel: [w282] -> w178 mode=indexing
        n43 = Initialize Array(0.0 ("Element"), w287) -> (w285:dbl[])
        n44 = Initialize Array(FALSE, w287) -> (w283:bool[])
        n45 = Bundle(w285) -> (w284:cluster{dbl[]})  [unwired: 1 in]
        n46 = Bundle(w283) -> (w282:cluster{bool[]})  [unwired: 1 in]
      }
      n47 = Bundle("DIOsMod0Name"=w126, "DIOsMod1Name"=w127, "DIOsMod2AName"=w125, "DIOsMod2BName"=w124, "ReglerNameMod0"=w139, "ReglerNameMod1"=w138, "ReglerNameMod2A"=w137, "ReglerNameMod2B"=w136, "LangsameHeizungen"=w207) -> (w269:T6)  [unwired: 1 in]
      n48 = Build Array (concatenate)(w139, w138, w137, w136) -> (w161:string[])
      n49 = Build Array (concatenate)(w229, w228, w227, w226) -> (w280:string[])
      n50 = Build Array (concatenate)(w233, w232, w231, w230) -> (w281:string[])
      n51 = Build Array (concatenate)(w225, w224, w223, w222) -> (w273:dbl[])
      n52 = Build Array (concatenate)(w221, w220, w219, w218) -> (w279:string[])
      n53 = Build Array (concatenate)(w139, w138, w137, w136) -> (→"HorstRegler":string[])
      n54 = Build Array (concatenate)(w96, w95, w94, w93) -> (w92:dbl[][])
      n55 = Array Size(array=w141) -> (size(s)=w77:i32)
      n56 = Build Array(w190, w189, w188, w187) -> (w186:i32[][])
      n57 = Array Size(array=w207) -> (size(s)=w206:i32)
      n58 = Add Array Elements(numeric array=w180) -> (sum=w265:i32)
      n59 = Array Size(array=w177) -> (size(s)=w176:i32)
      n60 = Index Array(array=w147, index=w146) -> (element=w145:T7)
      n61 = Add Array Elements(numeric array=w180) -> (sum=w192:i32)
      n62 = Decrement(x=w202) -> (x-1=w201:i32[])
      n63 = Build Cluster Array(w190, w189, w188, w187) -> (w272:cluster{"DIOsMod2BNr":i32[]}[])
      n64 = Build Array (concatenate)(w213, w212, w211) -> (w152:string[])
      n65 = Index Array(array=w214, index (col)=2 ("Deaktivierter Index (Spalte)")) -> (element=w261:dbl[])  [unwired: 1 in]
      n66 = Index Array(array=w214, index (col)=0 ("Deaktivierter Index (Spalte)")) -> (element=w259:dbl[])  [unwired: 1 in]
      n67 = Index Array(array=w214, index (col)=1 ("Deaktivierter Index (Spalte)")) -> (element=w260:dbl[])  [unwired: 1 in]
      n68 = Concatenate Strings("?SE0,SETP,0800" ("string"), "\n") -> (w103:string)
      n69 = Concatenate Strings("?SE0,SETP,2100" ("string"), "\n") -> (w110:string)
      n70 = Strip Path(path=w62) -> (stripped path=w61:path, name=w64:string)
      n71 = Concatenate Strings(w69, "Backup" ("string")) -> (w51:string)
      n72 = Build Path(base path=w66, name or relative path=w56) -> (appended path=w57:path)
      n73 = Build Path(base path=w67, name or relative path=w51) -> (appended path=w52:path)
      n74 = Concatenate Strings(w64, "Backup" ("string")) -> (w47:string)
      n75 = for {
        tunnel: w272 -> [w312] mode=indexing
        tunnel: [w313] -> w271 mode=indexing
        n76 = Unbundle(w312) -> ("DIOsMod2BNr"=w311:i32[])
        n77 = Array Size(array=w311) -> (size(s)=w313:i32)
      }
      n78 = property on="Methode" class="Ring (strikt)"("Strings []"=w274) -> ()  [unwired: 2 in, 2 out]
      n79 = Bundle("Modul1/AI sicherer Bereich"=w101, "Modul2/AI sicherer Bereich"=w100, "Modul3/AI sicherer Bereich"=w99, "Traps/Machs sicherer Bereich"=w98, w92, "Metavariablen grüner Bereich"=w91) -> (w97:T8)  [unwired: 1 in]
      n80 = Build Array (concatenate)(w174, w173) -> (w172:dbl[])
      n81 = Initialize Array(FALSE, w77) -> (w74:bool[])
      n82 = Array Size(array=w186) -> (size(s)=w185:i32[])
      n83 = Unbundle(w145) -> ("SPMPV"=w144:i32[])  [unwired: 44 out]
      n84 = Open/Create/Replace File(file path (use dialog)=path "c:/fromcriordy.txt" ("Dateipfad (Dialog verwenden)"), operation (0:open)=T4."replace or create" ("Operation (0:Öffnen)")) -> (refnum out=w238:refnum<file>, error out=w239:errorcluster)  [unwired: 4 in, 1 out]
      n85 = Initialize Array(0.0 ("element"), w77) -> (w75:dbl[])
      n86 = Initialize Array(0.0 ("Element"), w192) -> (w191:dbl[])
      n87 = Build Path(base path=w61, name or relative path=w47) -> (appended path=w46:path)
      n88 = Get Date/Time In Seconds() -> (seconds since 1Jan1904=w134:timestamp)
      n89 = Initialize Array(FALSE, w176) -> (w171:bool[])
      n90 = Multiply(x=w201, y=32) -> (x*y=w204:i32[])
      n91 = Initialize Array(-1.0, w192) -> (w194:dbl[])
      n92 = Array Subset(array=w152, index=32 ("Index"), length=32 ("Länge")) -> (→"AIs2":string[])
      n93 = Array Subset(array=w152, index=0 ("Index"), length=32 ("Länge")) -> (→"AIs1":string[])
      n94 = Array Subset(array=w152, index=64 ("Index"), length=32 ("Länge")) -> (→"AIs3":string[])
      n95 = global write "GVHK1Hz_ECD.vi" "Mod1Mod2Mod3/AITrapsMachs1Hz"(w172) -> ()
      n96 = global write "GVMetavariablen_ECD.vi" "Metavariablen"(w75) -> ()
      n97 = global write "GVHeizenLH_ECD.vi" "Heizen?LH"(w171) -> ()
      n98 = global write "GVZwangs_ECD.vi" "ZwangsLangsameHeizungenAn!"(w171) -> ()
      n99 = for {
        tunnel: w185 -> [w292] mode=indexing
        tunnel: [w289] -> w184 mode=indexing
        n100 = Initialize Array(FALSE, w292) -> (w290:bool[])
        n101 = Bundle(w290) -> (w289:cluster{bool[]})  [unwired: 1 in]
      }
      n102 = global write "GVHorstSP_ECD.vi" "HorstSP"(w191) -> ()
      n103 = global write "GVZwangs_ECD.vi" "ZwangsLangsameHeizungenAn?"(w171) -> ()
      n104 = global write "GVMetavariablen_ECD.vi" "MVFixwert"(w75) -> ()
      n105 = Add(x=w204, y=w177) -> (x+y=w203:i32[])
      n106 = Close File(refnum=w238, error in=w239) -> (path=w270:path)  [unwired: 1 out]
      n107 = Format Date/Time String(time format string (%c)="%Y-%m-%d--%H-%M" ("Zeitformatierungs-String (%c)"), seconds (now)=w134) -> (date/time string=w48:string)  [unwired: 1 in]
      n108 = Concatenate Strings(w51, w48) -> (w53:string)
      n109 = Concatenate Strings(w47, w48) -> (w49:string)
      n110 = Build Path(base path=w52, name or relative path=w53) -> (appended path=w50:path)
      n111 = Build Path(base path=w46, name or relative path=w49) -> (appended path=w45:path)
      n112 = Concatenate Strings(w56, w48) -> (w55:string)
      n113 = Create Folder(path (use dialog)=w50) -> (created path=w59:path)  [unwired: 2 in, 2 out]
      n114 = Create Folder(path (use dialog)=w45) -> (created path=w58:path)  [unwired: 2 in, 2 out]
      n115 = Bundle("created path"=w59, "created path"=w58) -> (w60:T9)  [unwired: 1 in]
      n116 = String To Byte Array(string=w103) -> (unsigned byte array=w105:u8[])
      n117 = String To Byte Array(string=w110) -> (unsigned byte array=w115:u8[])
      n118 = global write "GVMetavariablen_ECD.vi" "MVFix?"(w74) -> ()
      n119 = Index Array(array=w144, index=0) -> (element=w142:i32)
      n120 = Build Path(base path=w57, name or relative path=w55) -> (appended path=w54:path)
      n121 = call "FPGA-Start_ECD.vi"() -> ("error out"=w89:errorcluster, "FPGA-VI-Referenz (Ausgang)"=w88:refnum<k20>)  [unwired: 2 in]
      n122 = local write "MVFix?"(w74) -> ()
      n123 = local write "MVFixwert"(w75) -> ()
      n124 = global write "GVMWHorst_ECD.vi" "MWHorst"(w194) -> ()
      n125 = global write "GVVentilposition_ECD.vi" "Ventilposition"(w142) -> ()
      n126 = Build Array (concatenate)(string[] ["Jahr", "Monat", "Tag", "Stunde", "Minute", "Sekunde"] ("Array"), string[] ["Datei Nr.", "Methode Nr.", "Zyklusnr. Mod0", "Zyklusnr. Mod1", "Zyklusnr. Mod2A", "Zyklusnr. Mod2B"], w276, w152, w78, w161, "Probenvolumen1", "Probenvolumen2", "Ventilposition" ("element"), string[] ["CPU Total", "CPU Time critical", "CPU Timed Structures", "CPU High", "CPU Above normal", "CPU Normal", "CPU Background", "CPU Idle", "CPU ISR", "Memory", "SekundenTotalBrutal"]) -> (w278:string[])
      n127 = Build Array (concatenate)(w78, w161) -> (w160:string[])
      n128 = Build Array (concatenate)(w152, w78, w161) -> (w159:string[])
      n129 = Join Numbers(hi=w105, lo=u8 5) -> ((hi.lo)=w102:u16[])
      n130 = Join Numbers(hi=w115, lo=u8 6) -> ((hi.lo)=w113:u16[])
      n131 = Split 1D Array(array=w276, index=2 ("Index")) -> (second subarray=w268:string[])  [unwired: 1 out]
      n132 = Concatenate Strings("HK " ("String"), w48) -> (w121:string)
      n133 = Concatenate Strings("ECD1 " ("String"), w48) -> (w119:string)
      n134 = Concatenate Strings("ECD2 " ("String"), w48) -> (w117:string)
      n135 = property on="dargestellte Größe 1" class="Ring (strikt)"("Strings []"=w159) -> ()  [unwired: 2 in, 2 out]
      n136 = global write "GVZwangs_ECD.vi" "ZwangsHorst!"(w179) -> ()
      n137 = global write "GVZwangs_ECD.vi" "ZwangsHorst?"(w178) -> ()
      n138 = xnode "Invoke Method"("FPGA-VI-Referenz (Eingang)"=w88, "Daten"=w102) -> ("FPGA-VI-Referenz (Ausgang)"=w108:refnum<k20>)  [unwired: 2 in, 2 out]
      n139 = property on="dargestellte Größe 2" class="Ring (strikt)"("Strings []"=w159) -> ()  [unwired: 2 in, 2 out]
      n140 = property on="dargestellte Größe 3" class="Ring (strikt)"("Strings []"=w160) -> ()  [unwired: 2 in, 2 out]
      n141 = property on="Zeitachse2" class="Ring (strikt)"("Strings []"=w268) -> ()  [unwired: 2 in, 2 out]
      n142 = property on="Zeitachse1" class="Ring (strikt)"("Strings []"=w268) -> ()  [unwired: 2 in, 2 out]
      n143 = xnode "Invoke Method"("FPGA-VI-Referenz (Eingang)"=w108, "Daten"=w113) -> ("FPGA-VI-Referenz (Ausgang)"=w44:refnum<k20>)  [unwired: 2 in, 2 out]
      n144 = Create Folder(path (use dialog)=w54) -> (created path=w71:path)  [unwired: 2 in, 2 out]
      n145 = Build Path(base path=w65, name or relative path=w121) -> (appended path=w80:path)
      n146 = Build Path(base path=w70, name or relative path=w119) -> (appended path=w131:path)
      n147 = Build Path(base path=w62, name or relative path=w117) -> (appended path=w133:path)
      n148 = global write "GVZwischenspeicher.vi" "read"(w43) -> ()
      n149 = global write "GVZwischenspeicher.vi" "write"(w43) -> ()
      n150 = Strip Path(path=w83) -> (name=w82:string)  [unwired: 1 out]
      n151 = global write "GVZwangs_ECD.vi" "ZwangsDIO!"(w184) -> ()
      n152 = global write "GVZwangs_ECD.vi" "ZwangsDIO?"(w184) -> ()
      n153 = call "MPVSenden_ECD.vi"("Ventilposition"=0, "FPGA-VI-Referenz (Ausgang) 2"=w44) -> ("FPGA-VI-Referenz (Ausgang)"=w86:refnum<k20>)  [unwired: 1 in, 2 out]
      n154 = Build Path(base path=w71, name or relative path=w82) -> (appended path=w73:path)
      n155 = Create Folder(path (use dialog)=w80) -> (created path=w84:path)  [unwired: 2 in, 2 out]
      n156 = Create Folder(path (use dialog)=w131) -> (created path=w130:path)  [unwired: 2 in, 2 out]
      n157 = Create Folder(path (use dialog)=w133) -> (created path=w132:path)  [unwired: 2 in, 2 out]
      n158 = Copy(10:w73, 11:w83) -> ()  [unwired: 3 in, 3 out]
      n159 = Strip Path(path=w79) -> (name=w81:string)  [unwired: 1 out]
      n160 = case shown="True" w148 {
        tunnel: [w303 w308] -> w252
        tunnel: [w303 w307] -> w251
        tunnel: w84 -> [_ w306]
        tunnel: w210 -> [_ w305]
        tunnel: w146 -> [_ w304]
        frame False {
          w303 = refnum<k34> refnum ("tdms1")
        }
        frame True {
          n161 = call "TDMS0_ECD.vi"("Startmethode"=w304, "Dateiname"=w305, "Dateiordner"=w306) -> ("tdms1"=w307:refnum<k34>, "tdms0"=w308:refnum<k34>)
          n162 = global write "GVaktuelleTDMS_ECD.vi" "aktuelleTDMS-DateiHK"(w308) -> ()
        }
      }
      n163 = case shown="True" w148 {
        tunnel: [w293 w302] -> w250
        tunnel: [w293 w301] -> w249
        tunnel: [w293 w300] -> w248
        tunnel: [w293 w299] -> w247
        tunnel: w130 -> [_ w298]
        tunnel: w209 -> [_ w297]
        tunnel: w132 -> [_ w296]
        tunnel: w208 -> [_ w295]
        tunnel: w146 -> [_ w294]
        frame False {
          w293 = refnum<k34> refnum ("tdms0")
        }
        frame True {
          n164 = call "TDMS0_ECD.vi"("Startmethode"=w294, "Dateiname"=w297, "Dateiordner"=w298) -> ("tdms1"=w301:refnum<k34>, "tdms0"=w302:refnum<k34>)
          n165 = call "TDMS0_ECD.vi"("Startmethode"=w294, "Dateiname"=w295, "Dateiordner"=w296) -> ("tdms1"=w299:refnum<k34>, "tdms0"=w300:refnum<k34>)
          n166 = global write "GVaktuelleTDMS_ECD.vi" "aktuelleTDMS-DateiECD1"(w302) -> ()
          n167 = global write "GVaktuelleTDMS_ECD.vi" "aktuelleTDMS-DateiECD2"(w300) -> ()
        }
      }
      n168 = Build Path(base path=w71, name or relative path=w81) -> (appended path=w72:path)
      n169 = Copy(10:w72, 11:w79) -> ()  [unwired: 3 in, 3 out]
      n170 = Open/Create/Replace File(file path (use dialog)=path "c:/fromcriocmd.txt" ("Pfad MS-Datei CRIO"), operation (0:open)=T4."replace or create" ("Operation (0:Öffnen)")) -> (refnum out=w244:refnum<file>, error out=w243:errorcluster)  [unwired: 4 in, 1 out]
      n171 = Write to Text File(file (use dialog)=w244, text="time=yyyymmddhhmmss\ncycle=005\ninfo=1234567890123456789012345678901234567890123456789012345678901234567890123456789012345678901234567890\nlength=100\ncmd=cycle" ("Text0 MS-Datei"), error in=w243) -> (refnum out=w241:refnum<file>, error out=w240:errorcluster)  [unwired: 1 in, 1 out]
      n172 = Bundle("created path"=w84, "created path"=w130, "created path"=w132, "Dateiname Housekeeping"=w210, "DateinameECD1"=w209, "DateinameECD2"=w208, "tdms0"=w252, "tdms1"=w251, "tdms0"=w250, "tdms1"=w249, "tdms0"=w248, "tdms1"=w247) -> (w253:T10)  [unwired: 1 in]
      n173 = call "AIKoeffSortieren_ECD.vi"("Modul3/AI koeff"=w215, "Modul2/AI koeff"=w216, "Modul1/AI koeff"=w217) -> ("P0"=w256:dbl[], "P1"=w257:dbl[], "P2"=w258:dbl[])
      n174 = Close File(refnum=w241, error in=w240) -> (path=w235:path)  [unwired: 1 out]
      "schnelle Heizungen" <- w78
    }
    frame #1 {
      w323 = dbl[] [-1.0]
      w394 = 0
      w369 = 0 ("Zyklusnummer1")
      n175 = Add Array Elements(numeric array=w343) -> (sum=w342:i32)
      n176 = Array Size(array=w351) -> (size(s)=w372:i32)
      n177 = Unbundle(w368) -> ("created path"=w367:path, "created path"=w365:path, "created path"=w364:path, "Dateiname Housekeeping"=w366:string, "DateinameECD1"=w363:string, "DateinameECD2"=w362:string, "tdms0"=w361:refnum<k34>, "tdms1"=w360:refnum<k34>, "tdms0"=w359:refnum<k34>, "tdms1"=w358:refnum<k34>, "tdms0"=w357:refnum<k34>, "tdms1"=w356:refnum<k34>)
      n178 = Index Array(array=w344, index #1=0 ("Index"), index #2=1 ("Index"), index #3=2 ("Index"), index #4=3 ("Index")) -> (element #1=w383:i32, element #2=w382:i32, element #3=w385:i32, element #4=w384:i32)
      n179 = while {
        shift-right: ["Methode"] -> _
        shift-left: w420 -> [w1207]
        stop <- w1209 stop-if-true
        n180 = call "Bis zum nächsten Vielfachen warten7"("Count(mSec)"=u32 1000) -> ()  [unwired: 1 out]
        n181 = Not Equal?(x=w1207, y="Methode") -> (x != y?=w1205:bool)
        n182 = global read "gvbooleschRT_ECD.vi" "global stop RT"() -> (w1209:bool)
        n183 = global write "GVMethodenwechsel_ECD.vi" "Methodenwechsel?"(w1205) -> ()
      }
      n184 = call <vilib>:"Space Constant.vi"() -> ("String"=w329:string)
      n185 = while {
        tunnel: w347 -> [w654]
        tunnel: w416 -> [w657]
        tunnel: w415 -> [w656]
        tunnel: w414 -> [w655]
        shift-right: [w659] -> _
        shift-left: errorcluster {"status"=FALSE, "code"=0, "source"=""} ("error out") -> [w658]
        stop <- w660 stop-if-true
        n186 = call "AIsFIFORT_ECD.vi"("FPGA-VI-Referenz (Ausgang)"=w654, "P2"=w657, "P1"=w656, "P0"=w655, "error in"=w658) -> ("error out"=w659:errorcluster)
        "AIsFIFOread" <- w659
        n187 = global read "gvbooleschRT_ECD.vi" "global stop RT"() -> (w660:bool)
      }
      n188 = while {
        tunnel: w347 -> [w661]
        tunnel: w322 -> [w664]
        tunnel: w321 -> [w663]
        tunnel: w320 -> [w662]
        shift-right: [w666] -> _
        shift-left: errorcluster {"status"=FALSE, "code"=0, "source"=""} ("error out") -> [w665]
        stop <- w668 stop-if-true
        n189 = call "Bis zum nächsten Vielfachen warten16"("Count(mSec)"=u32 100) -> ()  [unwired: 1 out]
        n190 = call "TrapsMachMitteln_ECD.vi"("FPGA-VI-Referenz (Ausgang)"=w661, "Traps/MachKoeff2"=w664, "Traps/MachKoeff1"=w663, "Traps/MachKoeff0"=w662, "error in"=w665) -> ("error out"=w666:errorcluster)
        "MWTrapsMachs" <- w666
        n191 = global read "gvbooleschRT_ECD.vi" "global stop RT"() -> (w668:bool)
      }
      n192 = for {
        N: 1 -> [_]
        tunnel: w347 -> [w669]
        tunnel: [w669] -> w374
        n193 = call "Warten8"("Count(mSec)"=u32 100) -> ()  [unwired: 1 out]
      }
      n194 = Build Array(w329) -> (w328:string[])
      n195 = Initialize Array(-1 ("Element"), 4 ("Dimension")) -> (w345:i32[])
      n196 = global read "GVVentilposition_ECD.vi" "Ventilposition"() -> (w353:i32)
      n197 = Add(x=w385, y=w384) -> (x+y=w381:i32)
      n198 = Bundle(w328, w328, w328) -> (w392:cluster{string[], string[], string[]})  [unwired: 1 in]
      n199 = Index Array(array=w338, index=w336) -> (element=w337:T7)
      n200 = Initialize Array(cluster{"output high":dbl, "output low":dbl} {"output high"=99999.0, "output low"=0.0} ("output range"), w372) -> (w352:cluster{"output high":dbl, "output low":dbl}[])
      n201 = while {
        tunnel: w419 -> [w785]
        shift-right: [w784] -> _
        shift-left: w338 -> [w766]
        tunnel: w352 -> [w783]
        tunnel: w351 -> [w782]
        tunnel: w347 -> [w781]
        tunnel: w350 -> [w780]
        tunnel: w349 -> [w779]
        shift-right: [w773] -> _
        shift-left: 0 -> [w778]
        tunnel: w347 -> [w777]
        tunnel: w346 -> [w776]
        shift-right: [w772] -> _
        shift-left: w345 -> [w775]
        tunnel: w344 -> [w767]
        tunnel: w343 -> [w768]
        tunnel: w342 -> [w769]
        tunnel: w341 -> [w770]
        tunnel: w340 -> [w771]
        tunnel: w339 -> [w774]
        shift-right: [w690] -> _
        shift-left: w337 -> [w689]
        tunnel: w322 -> [w675]
        tunnel: w321 -> [w676]
        tunnel: w320 -> [w677]
        tunnel: w315 -> [w678]
        tunnel: w314 -> [w674]
        i -> [w693]
        stop <- w786 stop-if-true
        w683 = 0  # ZeileMainMach2
        w684 = 0  # ZeileMainMach1
        w734 = FALSE
        w733 = 0.0
        w735 = 0  # ZeilennummerMPV
        w739 = cluster{dbl[], dbl[]} {[], []}
        w748 = dbl[] []
        w752 = 0  # ZeilePreMach2
        w753 = 0  # ZeilePreMach1
        w754 = 0  # ZeileFPGAFixp
        w755 = 0  # ZeileFPGAPID
        w756 = 0  # ZeileFPGABoolesch
        w757 = i32[] [0, 0, 0, 0]  # ZeilennummernHorst
        w758 = i32[] [0, 0, 0, 0]  # ZeilennummernDIOs
        n202 = Unbundle(w674) -> ("created path"=w673:path, "created path"=w672:path)
        n203 = Unbundle(w689) -> ("Zykluslängen [s]"=w671:dbl[], "ZeitpktDIOsMod0"=w732:dbl[], "ZeitpktDIOsMod1"=w731:dbl[], "ZeitpktDIOsMod2A"=w730:dbl[], "ZeitpktDIOsMod2B"=w729:dbl[], "DIOsSPMod0"=w728:bool[][], "DIOsSPMod1"=w727:bool[][], "DIOsSPMod2A"=w726:bool[][], "DIOsSPMod2B"=w725:bool[][], "Mod0HorstZeitpkt"=w724:dbl[], "Mod1HorstZeitpkt"=w723:dbl[], "Mod2AHorstZeitpkt"=w722:dbl[], "Mod2BHorstZeitpkt"=w721:dbl[], "HorstSPMod0"=w720:dbl[][], "HorstSPMod1"=w719:dbl[][], "HorstSPMod2A"=w718:dbl[][], "HorstSPMod2B"=w717:dbl[][], "LHSetpoints"=w716:dbl[], "LHHeizen?"=w715:bool[], "ZPktFPGABoolesch"=w714:dbl[], "FPGABoolesch"=w713:bool[][], "ZeitpktFPGAPID"=w712:dbl[], "FPGAPID"=w711:T11, "ZeitpktFPGAFixp"=w710:dbl[], w709:dbl[][], "t_PreMach1"=w708:dbl[], "T_PreMach1"=w707:dbl[], "t_PreMach2"=w706:dbl[], "T_PreMach2"=w705:dbl[], "PIDs für \"träge\" Heizungen"=w704:T12, "Zwangsbedingungen"=w703:dbl[][], "Dateien fürs MS schicken?"=w702:bool, "ZeitpunkteMPV"=w701:dbl[], "SPMPV"=w700:i32[], "ZeitpktMS-1"=w699:dbl, "ZeitpktMS-2"=w698:dbl, "Int.Start1"=w697:dbl, "Int.Stop1"=w696:dbl, "Int.Start2"=w695:dbl, "Int.Stop2"=w694:dbl, "t_MainMach1"=w688:dbl[], "T_MainMach1"=w687:dbl[], "t_MainMach2"=w686:dbl[], "T_MainMach2"=w685:dbl[])  [unwired: 1 out]
        n204 = while {
          tunnel: w671 -> [w819]
          tunnel: w672 -> [w809]
          stop <- w808 stop-if-true
          n205 = global read "GVZeitenZyklen_ECD.vi" "Big Ben, Methodenzeit, Zykluszeit0, Zykluszeit1, Zykluszeit2A, Zykluszeit2B"() -> (w817:dbl[])
          n206 = Index Array(array=w817, index=5) -> (element=w815:dbl)
          n207 = global read "GVZeitenZyklen_ECD.vi" "ZyklusNummernGesamt"() -> (w820:i32[])
          n208 = call "Wait Until Next Multiple2"("Count(mSec)"=u32 100) -> ()  [unwired: 1 out]
          n209 = Index Array(array=w819, index=3) -> (element=w814:dbl)
          n210 = Subtract(x=w814, y=0.2) -> (x-y=w812:dbl)
          n211 = Greater Or Equal?(x=w815, y=w812) -> (x >= y?=w811:bool)
          n212 = global read "GVChroms_ECD.vi" "ECD2Chrom"() -> (w810:dbl[])
          n213 = case shown="True" w811 {
            tunnel: w820 -> [_ w828]
            tunnel: w810 -> [_ w827]
            tunnel: w809 -> [_ w826]
            frame False {
            }
            frame True {
              n214 = flat-sequence {
                tunnel: w828 -> [w844]
                tunnel: w827 -> [w831]
                tunnel: w826 -> [w830]
                frame #0 {
                  n215 = Index Array(array=w844, index=3) -> (element=w842:i32)
                  n216 = Number To Decimal String(number=w842, width (-)=i16 4) -> (decimal integer string=w840:string)
                  n217 = Concatenate Strings(w840, "ECD2.hag" ("string")) -> (w838:string)
                  n218 = Build Path(base path=w830, name or relative path=w838) -> (appended path=w829:path)
                  n219 = Open/Create/Replace File(file path (use dialog)=w829, operation (0:open)=T4."replace or create") -> (refnum out=w837:refnum<file>, error out=w836:errorcluster)  [unwired: 4 in, 1 out]
                  n220 = Write to Binary File(file (use dialog)=w837, data=w831, error in=w836) -> (refnum out=w835:refnum<file>, error out=w834:errorcluster)  [unwired: 3 in, 1 out]
                  n221 = Close File(refnum=w835, error in=w834) -> (error out=→"ECD2dataBackup":errorcluster)  [unwired: 1 out]
                }
                frame #1 {
                  n222 = call "Wait2"("Count(mSec)"=u32 2000) -> ()  [unwired: 1 out]
                }
              }
            }
          }
          n223 = global read "GVMethodenwechsel_ECD.vi" "Methodenwechsel?"() -> (w823:bool)
          n224 = global read "gvbooleschRT_ECD.vi" "global stop RT"() -> (w824:bool)
          n225 = Or(x=w823, y=w824) -> (x .or. y?=w825:bool)
          n226 = local read "veränderte Methode benutzen"() -> (w822:bool)
          n227 = Or(x=w825, y=w822) -> (x .or. y?=w808:bool)
        }
        n228 = while {
          tunnel: w671 -> [w856]
          tunnel: w673 -> [w846]
          stop <- w860 stop-if-true
          n229 = global read "GVZeitenZyklen_ECD.vi" "Big Ben, Methodenzeit, Zykluszeit0, Zykluszeit1, Zykluszeit2A, Zykluszeit2B"() -> (w854:dbl[])
          n230 = Index Array(array=w854, index=4) -> (element=w852:dbl)
          n231 = global read "GVZeitenZyklen_ECD.vi" "ZyklusNummernGesamt"() -> (w857:i32[])
          n232 = call "Wait Until Next Multiple"("Count(mSec)"=u32 100) -> ()  [unwired: 1 out]
          n233 = Index Array(array=w856, index=2) -> (element=w851:dbl)
          n234 = Subtract(x=w851, y=0.2) -> (x-y=w849:dbl)
          n235 = Greater Or Equal?(x=w852, y=w849) -> (x >= y?=w848:bool)
          n236 = global read "GVChroms_ECD.vi" "ECD1Chrom"() -> (w847:dbl[])
          n237 = case shown="True" w848 {
            tunnel: w857 -> [_ w866]
            tunnel: w847 -> [_ w865]
            tunnel: w846 -> [_ w864]
            frame False {
            }
            frame True {
              n238 = flat-sequence {
                tunnel: w866 -> [w882]
                tunnel: w865 -> [w869]
                tunnel: w864 -> [w868]
                frame #0 {
                  n239 = Index Array(array=w882, index=2) -> (element=w880:i32)
                  n240 = Number To Decimal String(number=w880, width (-)=i16 4) -> (decimal integer string=w878:string)
                  n241 = Concatenate Strings(w878, "ECD1.hag" ("string")) -> (w876:string)
                  n242 = Build Path(base path=w868, name or relative path=w876) -> (appended path=w867:path)
                  n243 = Open/Create/Replace File(file path (use dialog)=w867, operation (0:open)=T4."replace or create") -> (refnum out=w875:refnum<file>, error out=w874:errorcluster)  [unwired: 4 in, 1 out]
                  n244 = Write to Binary File(file (use dialog)=w875, data=w869, error in=w874) -> (refnum out=w873:refnum<file>, error out=w872:errorcluster)  [unwired: 3 in, 1 out]
                  n245 = Close File(refnum=w873, error in=w872) -> (error out=→"ECD1dataBackup":errorcluster)  [unwired: 1 out]
                }
                frame #1 {
                  n246 = call "Wait"("Count(mSec)"=u32 2000) -> ()  [unwired: 1 out]
                }
              }
            }
          }
          n247 = global read "GVMethodenwechsel_ECD.vi" "Methodenwechsel?"() -> (w861:bool)
          n248 = global read "gvbooleschRT_ECD.vi" "global stop RT"() -> (w862:bool)
          n249 = Or(x=w861, y=w862) -> (x .or. y?=w863:bool)
          n250 = local read "veränderte Methode benutzen"() -> (w859:bool)
          n251 = Or(x=w863, y=w859) -> (x .or. y?=w860:bool)
        }
        n252 = Add(x=w775, y=1) -> (x+y=w743:i32[])
        n253 = local read "Methode"() -> (w692:i32)
        n254 = Build Cluster Array(w728, w727, w726, w725) -> (w762:cluster{"DIOsSPMod2B":bool[][]}[])
        n255 = Build Cluster Array(w720, w719, w718, w717) -> (w760:cluster{"HorstSPMod2B":dbl[][]}[])
        n256 = Build Cluster Array(w732, w731, w730, w729) -> (w763:cluster{"ZeitpktDIOsMod2B":dbl[]}[])
        n257 = Build Cluster Array(w724, w723, w722, w721) -> (w761:cluster{"Mod2BHorstZeitpkt":dbl[]}[])
        n258 = Equal?(x=w693, y=0) -> (x = y?=w764:bool)
        n259 = while {
          tunnel: w671 -> [w794]
          stop <- w797 stop-if-true
          n260 = global read "GVZeitenZyklen_ECD.vi" "Big Ben, Methodenzeit, Zykluszeit0, Zykluszeit1, Zykluszeit2A, Zykluszeit2B"() -> (w803:dbl[])
          n261 = To Long Integer(number="Zyklus") -> (32bit integer=w789:i32)
          n262 = Index Array(array=w794, index=w789) -> (element=w793:dbl)
          n263 = Subtract(x=w793, y=1.0) -> (x-y=w791:dbl)
          n264 = Add(x=w789, y=2) -> (x+y=w787:i32)
          n265 = call "Wait3"("Count(mSec)"=u32 100) -> ()  [unwired: 1 out]
          n266 = global read "GVMethodenwechsel_ECD.vi" "Methodenwechsel?"() -> (w799:bool)
          n267 = global read "gvbooleschRT_ECD.vi" "global stop RT"() -> (w800:bool)
          n268 = local read "am Ende benutzen"() -> (w802:bool)
          n269 = local read "veränderte Methode benutzen"() -> (w795:bool)
          n270 = Index Array(array=w803, index=w787) -> (element=w804:dbl)
          n271 = Or(x=w799, y=w800) -> (x .or. y?=w798:bool)
          n272 = Greater Or Equal?(x=w804, y=w791) -> (x >= y?=w805:bool)
          n273 = And(x=w805, y=w802) -> (x .and. y?=w796:bool)
          n274 = case shown="True" w796 {
            frame False {
            }
            frame True {
              n275 = local write "veränderte Methode benutzen"(TRUE ("veränderte Methode benutzen")) -> ()
              n276 = local write "am Ende benutzen"(FALSE ("am Ende benutzen")) -> ()
            }
          }
          n277 = Or(x=w798, y=w795) -> (x .or. y?=w797:bool)
        }
        n278 = while {
          tunnel: w768 -> [w952]
          tunnel: w771 -> [w945]
          tunnel: w770 -> [w946]
          tunnel: w767 -> [w951]
          tunnel: w769 -> [w947]
          tunnel: w703 -> [w948]
          stop <- w954 stop-if-true
          n279 = call "Bis zum nächsten Vielfachen warten10"("Count(mSec)"=u32 1000) -> ()  [unwired: 1 out]
          n280 = local read "Methode"() -> (w950:i32)
          n281 = global read "GVMethodenwechsel_ECD.vi" "Methodenwechsel?"() -> (w956:bool)
          n282 = global read "gvbooleschRT_ECD.vi" "global stop RT"() -> (w957:bool)
          n283 = case shown="True" "global stop RT" {
            frame False {
            }
            frame True {
              n284 = global write "gvbooleschRT_ECD.vi" "global stop RT"(TRUE ("global stop RT")) -> ()
            }
          }
          n285 = call "ZwangsbedingungenGV_ECD.vi"("AnzahlHorst"=w945, "AnzahlHorst/Modul"=w951, "AnzahlLH"=w946, "AnzahlDIOs/Modul"=w952, "AnzahlDIOs"=w947, "Zwangsbedingungen"=w948, "Methodennummer"=w950) -> ("Methodennummer"=w949:i32)  [unwired: 4 in]
          n286 = local write "Methode"(w949) -> ()
          n287 = local read "veränderte Methode benutzen"() -> (w955:bool)
          n288 = Compound Arithmetic op=OR(w957, w956, w955) -> (w954:bool)
        }
        n289 = global read "GVZeitenZyklen_ECD.vi" "ZyklusNummern"() -> (w742:i32[])
        n290 = global read "GVZwangs_ECD.vi" "ZwangsHorst?"() -> (w747:cluster{bool[]}[])
        n291 = global read "gvbooleschRT_ECD.vi" "global stop RT"() -> (w786:bool)
        n292 = global read "GVZwangsMPV_ECD.vi" "ZwangsMPV?"() -> (w681:bool)
        n293 = global read "GVZwangs_ECD.vi" "ZwangsDIO?"() -> (w746:cluster{bool[]}[])
        n294 = global read "GVaktuelleTDMS_ECD.vi" "aktuelleTDMS-DateiECD1"() -> (w741:refnum<k34>)
        n295 = Bundle(w763, w762, w761, w760, "LHHeizen?"=w715, "ZPktFPGABoolesch"=w714, "FPGABoolesch"=w713, "ZeitpktFPGAPID"=w712, "FPGAPID"=w711, "ZeitpktFPGAFixp"=w710, w709, "t_PreMach1"=w708, "T_PreMach1"=w707, "t_PreMach2"=w706, "T_PreMach2"=w705, "ZeitpunkteMPV"=w701, "SPMPV"=w700, "t_MainMach1"=w688, "T_MainMach1"=w687, "t_MainMach2"=w686, "T_MainMach2"=w685) -> (w759:T13)  [unwired: 1 in]
        n296 = Index Array(array=w766, index=w692) -> (element=w691:T7)
        n297 = global read "GVZwangs_ECD.vi" "ZwangsFPGABoolesch?"() -> (w745:bool[])
        n298 = while {
          tunnel: w782 -> [w935]
          tunnel: w783 -> [w938]
          tunnel: w781 -> [w939]
          tunnel: w716 -> [w936]
          tunnel: w704 -> [w937]
          shift-right: [w933] -> _
          shift-left: errorcluster {"status"=FALSE, "code"=0, "source"=""} ("error out") -> [w934]
          stop <- w940 stop-if-true
          n299 = call "LH_ECD.vi"("FPGA-VI-Referenz (Ausgang)"=w939, "OutputRange"=w938, "LHSetpoints"=w936, "AIsLH"=w935, "error in"=w934, "LH-Gruppe"="LH-Gruppe", "PIDs für \"träge\" Heizungen"=w937) -> ("error out"=w933:errorcluster)
          "LH" <- w933
          n300 = call "Bis zum nächsten Vielfachen warten12"("Count(mSec)"=u32 100) -> ()  [unwired: 1 out]
          n301 = global read "GVMethodenwechsel_ECD.vi" "Methodenwechsel?"() -> (w942:bool)
          n302 = global read "gvbooleschRT_ECD.vi" "global stop RT"() -> (w943:bool)
          n303 = local read "veränderte Methode benutzen"() -> (w941:bool)
          n304 = Compound Arithmetic op=OR(w943, w942, w941) -> (w940:bool)
        }
        n305 = while {
          shift-right: [w896] -> _
          shift-left: w734 -> [w900]
          shift-right: [w895] -> _
          shift-left: w733 -> [w899]
          shift-right: [w894] -> _
          shift-left: w734 -> [w898]
          shift-right: [w893] -> _
          shift-left: w733 -> [w897]
          tunnel: w774 -> [w892]
          tunnel: w697 -> [w887]
          tunnel: w696 -> [w886]
          tunnel: w695 -> [w885]
          tunnel: w694 -> [w884]
          stop <- w889 stop-if-true
          n306 = call "Integrieren_ECD.vi"("Integrieren1"=w900, "Integral1"=w899, "Integrieren2"=w898, "Integral2"=w897, "Int.Start1"=w887, "Int.Stop1"=w886, "Int.Start2"=w885, "HorstProbenflußNr."=w892, "Int.Stop2"=w884) -> ("Integrieren1"=w896:bool, "Integral1"=w895:dbl, "Integrieren2"=w894:bool, "Integral2"=w893:dbl)  [unwired: 7 in]
          n307 = call "Bis zum nächsten Vielfachen warten9"("Count(mSec)"=u32 100) -> ()  [unwired: 1 out]
          n308 = global read "GVMethodenwechsel_ECD.vi" "Methodenwechsel?"() -> (w890:bool)
          n309 = global read "gvbooleschRT_ECD.vi" "global stop RT"() -> (w891:bool)
          n310 = local read "veränderte Methode benutzen"() -> (w888:bool)
          n311 = Compound Arithmetic op=OR(w891, w890, w888) -> (w889:bool)
        }
        n312 = while "Zeit" {
          tunnel: w764 -> [w1144]
          tunnel: w671 -> [w1142]
          tunnel: w743 -> [w1137]
          tunnel: [w1136] -> w772
          shift-right: [w1133] -> _
          shift-left: 0.0 -> [w1134]
          i -> [w1146]
          stop <- w1139 stop-if-true
          n313 = Equal?(x=w1146, y=0) -> (x = y?=w1135:bool)
          n314 = call "Bis zum nächsten Vielfachen warten15"("Count(mSec)"=u32 50) -> ()  [unwired: 1 out]
          n315 = call "BigBen_ECD.vi"("MethodenStartzeit"=w1134, "Methodenstart?"=w1135, "Programmstart?"=w1144, "Zykluslängen [s]"=w1142, "MethodenStartZyklusNummern"=w1137) -> ("MethodenStartzeit"=w1133:dbl, "ZyklusNummernGesamt"=w1136:i32[])  [unwired: 2 in]
          n316 = global read "GVMethodenwechsel_ECD.vi" "Methodenwechsel?"() -> (w1138:bool)
          n317 = global read "gvbooleschRT_ECD.vi" "global stop RT"() -> (w1143:bool)
          n318 = Or(x=w1138, y=w1143) -> (x .or. y?=w1140:bool)
          n319 = local read "veränderte Methode benutzen"() -> (w1141:bool)
          n320 = Or(x=w1141, y=w1140) -> (x .or. y?=w1139:bool)
        }
        n321 = Bundle(w748, w748, w748, w748) -> (w749:cluster{dbl[], dbl[], dbl[], dbl[]})  [unwired: 1 in]
        n322 = while {
          tunnel: w785 -> [w1159]
          shift-right: [w1150] -> _
          shift-left: w691 -> [w1158]
          tunnel: w692 -> [w1156]
          shift-right: [w1148] -> w784
          shift-left: w766 -> [w1157]
          tunnel: [w1149] -> w690
          stop <- w1152 stop-if-true
          n323 = call "Bis zum nächsten Vielfachen warten8"("Count(mSec)"=u32 500) -> ()  [unwired: 1 out]
          n324 = global read "GVMethodenwechsel_ECD.vi" "Methodenwechsel?"() -> (w1154:bool)
          n325 = global read "gvbooleschRT_ECD.vi" "global stop RT"() -> (w1153:bool)
          n326 = case shown="True" "Methode verändern" {
            tunnel: w1159 -> [_ w1181]
            tunnel: w1158 -> [w1178 w1180]
            tunnel: [w1178 w1179] -> w1150
            frame False {
            }
            frame True {
              n327 = call "methodeändern_ECD.vi"("->Methode"=w1180, "Namen"=w1181) -> ("Methode->"=w1179:T14)  [unwired: 1 in]
              n328 = property on="Methode verändern" class="Bool. (strikt)"("Value"=FALSE ("Methode verändern")) -> ()  [unwired: 2 in, 2 out]
            }
          }
          n329 = Compound Arithmetic op=OR(w1154, w1153, "veränderte Methode benutzen") -> (w1152:bool)
          n330 = case shown="True" "Methode speichern" {
            tunnel: w1150 -> [_ w1175]
            tunnel: w1157 -> [w1168 w1177]
            tunnel: w1156 -> [_ w1176]
            tunnel: [w1168 w1170] -> w1148
            frame False {
            }
            frame True {
              n331 = Replace Array Subset(array=w1177, new element=w1175, index=w1176) -> (w1170:T2)
              n332 = property on="Methode speichern" class="Bool. (strikt)"("Value"=FALSE ("Methode speichern")) -> ()  [unwired: 2 in, 2 out]
              n333 = Open/Create/Replace File(file path (use dialog)=path "c:/methoden.pery" ("Dateipfad (Dialog verwenden)"), operation (0:open)=T4."replace" ("Operation (0:Öffnen)")) -> (refnum out=w1172:refnum<file>)  [unwired: 4 in, 2 out]
              n334 = Write to Binary File(file (use dialog)=w1172, data=w1170) -> (refnum out=w1169:refnum<file>)  [unwired: 4 in, 2 out]
              n335 = Close File(refnum=w1169) -> ()  [unwired: 1 in, 2 out]
            }
          }
          n336 = case shown="True" "veränderte Methode benutzen" {
            tunnel: w1150 -> [_ w1165]
            tunnel: [w1162 w1165] -> w1149
            tunnel: w1148 -> [w1164 _]
            frame False {
              n337 = local read "Methode"() -> (w1163:i32)
              n338 = Index Array(array=w1164, index=w1163) -> (element=w1162:T7)
            }
            frame True {
              n339 = flat-sequence {
                frame #0 {
                  n340 = call "Warten"("Count(mSec)"=u32 1100) -> ()  [unwired: 1 out]
                }
                frame #1 {
                  n341 = property on="veränderte Methode benutzen" class="Bool. (strikt)"("Value"=FALSE ("Methode verändern")) -> ()  [unwired: 2 in, 2 out]
                }
              }
            }
          }
        }
        n342 = Bundle("ZyklusNummern"=w742, "ZeilennummernDIOs"=w758, "ZwangsDIO?"=w746, "ZeilennummernHorst"=w757, "ZwangsHorst?"=w747, "ZeileFPGABoolesch"=w756, "ZwangsFPGABoolesch?"=w745, "ZeileFPGAPID"=w755, "ZeileFPGAFixp"=w754, "ZeilePreMach1"=w753, "ZeilePreMach2"=w752, "ZeilennummerMPV"=w735, "ZeileMainMach1"=w684, "ZeileMainMach2"=w683, "ZwangsMPV?"=w681) -> (w751:T15)  [unwired: 1 in]
        n343 = while {
          shift-right: [w1076] -> _
          shift-left: w749 -> [w1083]
          shift-right: [w1075] -> _
          shift-left: w749 -> [w1082]
          shift-right: [w1073] -> _
          shift-left: T5 {"Zyklus1"=0, "Zeitachse1"=0, "dargestellte Größe 1"=0, "Zyklus2"=0, "Zeitachse2"=0, "dargestellte Größe 2"=0} ("AnzeigeEinstellungen") -> [w1081]
          tunnel: w671 -> [w1051]
          shift-right: [w1047] -> _
          shift-left: w741 -> [w1046]
          shift-right: [w1042] -> _
          shift-left: w739 -> [w1044]
          shift-right: [w1031] -> _
          shift-left: w739 -> [w1043]
          shift-right: ["Detektor"] -> _
          shift-left: 0 ("Detektor") -> [w1040]
          tunnel: w678 -> [w1029]
          stop <- w1087 stop-if-true
          w1052 = 0.0 ("X-Achse.Bereich:Minimum")
          n344 = Unbundle(w1029) -> ("Modul1/AI sicherer Bereich"=w1022:dbl[][], "Modul2/AI sicherer Bereich"=w1007:dbl[][], "Modul3/AI sicherer Bereich"=w998:dbl[][], "Traps/Machs sicherer Bereich"=w989:dbl[][], w981:dbl[][], "Metavariablen grüner Bereich"=w972:dbl[][])
          n345 = call "Bis zum nächsten Vielfachen warten14"("Count(mSec)"=u32 1000) -> ()  [unwired: 1 out]
          n346 = global read "GVMWHorst_ECD.vi" "MWHorst"() -> (w980:dbl[])
          "MWHorst" <- w980
          n347 = case shown="0, Standard" "Detektor" {
            tunnel: [w1097 w1109] -> w1042
            tunnel: w1051 -> [w1096 w1111]
            tunnel: "Detektor" -> [w1091 w1105]
            tunnel: [w1095 w1110] -> w1049
            tunnel: [w1094 w1108] -> w1047
            frame 0, Default {
              n348 = Increment(x=w1091) -> (x+1=w1092:i32)
              n349 = Increment(x=w1092) -> (x+1=w1090:i32)
              n350 = global read "GVChroms_ECD.vi" "ECD1Chrom"() -> (w1093:dbl[])
              n351 = global read "GVaktuelleTDMS_ECD.vi" "aktuelleTDMS-DateiECD1"() -> (w1094:refnum<k34>)
              n352 = Index Array(array=w1096, index=w1090) -> (element=w1095:dbl)
              n353 = Array Size(array=w1093) -> (size(s)=w1099:i32)
              n354 = for {
                N: w1099 -> [_]
                tunnel: [w1100] -> w1098 mode=indexing
                i -> [w1103]
                n355 = To Double Precision Float(number=w1103) -> (double precision float=w1102:dbl)
                n356 = Divide(x=w1102, y=10.0) -> (x/y=w1100:dbl)
              }
              n357 = Bundle(w1098, "ECD1Chrom"=w1093) -> (w1097:cluster{dbl[], "ECD1Chrom":dbl[]})  [unwired: 1 in]
            }
            frame 1 {
              n358 = Increment(x=w1105) -> (x+1=w1106:i32)
              n359 = Increment(x=w1106) -> (x+1=w1104:i32)
              n360 = global read "GVChroms_ECD.vi" "ECD2Chrom"() -> (w1107:dbl[])
              n361 = global read "GVaktuelleTDMS_ECD.vi" "aktuelleTDMS-DateiECD2"() -> (w1108:refnum<k34>)
              n362 = Index Array(array=w1111, index=w1104) -> (element=w1110:dbl)
              n363 = Array Size(array=w1107) -> (size(s)=w1113:i32)
              n364 = for {
                N: w1113 -> [_]
                tunnel: [w1114] -> w1112 mode=indexing
                i -> [w1117]
                n365 = To Double Precision Float(number=w1117) -> (double precision float=w1116:dbl)
                n366 = Divide(x=w1116, y=10.0) -> (x/y=w1114:dbl)
              }
              n367 = Bundle(w1112, "ECD2Chrom"=w1107) -> (w1109:cluster{dbl[], "ECD2Chrom":dbl[]})  [unwired: 1 in]
            }
          }
          n368 = Subtract(x="DetYMax", y="DetYMin") -> (x-y=w1057:dbl)
          n369 = Subtract(x="HK1YMax", y="HK1YMin") -> (x-y=w1067:dbl)
          n370 = Subtract(x="HK2YMax", y="HK2YMin") -> (x-y=w1062:dbl)
          n371 = Equal?(x="Detektor", y=w1040) -> (x = y?=w1039:bool)
          n372 = Index Array(array=w1022, index (col) #1=0 ("disabled index (col)"), index (col) #2=1 ("index (col)")) -> (element #1=w1019:dbl[], element #2=w1017:dbl[])  [unwired: 2 in]
          n373 = Index Array(array=w1007, index (col) #1=0 ("disabled index (col)"), index (col) #2=1 ("index (col)")) -> (element #1=w1011:dbl[], element #2=w1010:dbl[])  [unwired: 2 in]
          n374 = Index Array(array=w989, index (col) #1=0 ("disabled index (col)"), index (col) #2=1 ("index (col)")) -> (element #1=w993:dbl[], element #2=w992:dbl[])  [unwired: 2 in]
          n375 = Index Array(array=w981, index (col) #1=0 ("disabled index (col)"), index (col) #2=1 ("index (col)")) -> (element #1=w985:dbl[], element #2=w984:dbl[])  [unwired: 2 in]
          n376 = Index Array(array=w998, index (col) #1=0 ("disabled index (col)"), index (col) #2=1 ("index (col)")) -> (element #1=w1002:dbl[], element #2=w1001:dbl[])  [unwired: 2 in]
          n377 = Index Array(array=w972, index (col) #1=0 ("disabled index (col)"), index (col) #2=1 ("index (col)")) -> (element #1=w976:dbl[], element #2=w975:dbl[])  [unwired: 2 in]
          n378 = call <vilib>:"RT Get CPU Loads.vi"() -> ("CPU loads"=w960:T16[])  [unwired: 10 in, 1 out]
          n379 = global read "GVMethodenwechsel_ECD.vi" "Methodenwechsel?"() -> (w1085:bool)
          n380 = global read "GVZeitenZyklen_ECD.vi" "ZyklusNummern"() -> (w1054:i32[])
          "ZyklusNummern" <- w1054
          n381 = global read "gvbooleschRT_ECD.vi" "global stop RT"() -> (w1086:bool)
          n382 = global read "GVMetavariablen_ECD.vi" "Metavariablen"() -> (w971:dbl[])
          "MVWerte" <- w971
          n383 = global read "GVVentilposition_ECD.vi" "Ventilposition"() -> (→"Ventilposition":i32)
          n384 = global read "GVZeitenZyklen_ECD.vi" "ZyklusNummernGesamt"() -> (→"ZyklusNummernGesamt":i32[])
          n385 = Divide(x=w1057, y=20.0) -> (x/y=w1055:dbl)
          n386 = Divide(x=w1067, y=10.0) -> (x/y=w1065:dbl)
          n387 = Divide(x=w1062, y=10.0) -> (x/y=w1060:dbl)
          n388 = Index Array(array=w960, index=0) -> (element=w964:T16)
          n389 = local read "veränderte Methode benutzen"() -> (w1084:bool)
          n390 = Or(x=w1085, y=w1086) -> (x .or. y?=w1088:bool)
          n391 = Greater Or Equal?(x=w980, y=w985) -> (x >= y?=w983:bool[])
          n392 = Less Or Equal?(x=w980, y=w984) -> (x <= y?=w982:bool[])
          n393 = Greater Or Equal?(x=w971, y=w976) -> (x >= y?=w974:bool[])
          n394 = Less Or Equal?(x=w971, y=w975) -> (x <= y?=w973:bool[])
          n395 = Unbundle(w964) -> ("Total (%)"=→"CPU Total (%)":dbl)  [unwired: 8 out]
          n396 = global read "GVHK1Hz_ECD.vi" "Mod1Mod2Mod3/AITrapsMachs1Hz"() -> (w967:dbl[])
          n397 = global write "GVMetavariablen_ECD.vi" "MVFixwert"("MVFixwert") -> ()
          n398 = And(x=w983, y=w982) -> (x .and. y?=→"HorstOK?":bool[])
          n399 = And(x=w974, y=w973) -> (x .and. y?=→"MVOK?":bool[])
          n400 = Or(x=w1088, y=w1084) -> (x .or. y?=w1087:bool)
          n401 = global write "GVMetavariablen_ECD.vi" "MVFix?"("MVFix?") -> ()
          n402 = global read "GVZeitenZyklen_ECD.vi" "Big Ben, Methodenzeit, Zykluszeit0, Zykluszeit1, Zykluszeit2A, Zykluszeit2B"() -> (w1034:dbl[])
          n403 = Array Subset(array=w967, index=0 ("Index"), length=32 ("Länge")) -> (w1018:dbl[])
          "AIs1" <- w1018
          n404 = Array Subset(array=w967, index=32 ("Index"), length=32 ("Länge")) -> (w1006:dbl[])
          "AIs2" <- w1006
          n405 = Array Subset(array=w967, index=96 ("Index"), length=6 ("Länge")) -> (w966:dbl[])
          "schnelle Heizungen" <- w966
          n406 = Array Subset(array=w967, index=64 ("Index"), length=32 ("Länge")) -> (w997:dbl[])
          "AIs3" <- w997
          n407 = Greater Or Equal?(x=w966, y=w993) -> (x >= y?=w991:bool[])
          n408 = Less Or Equal?(x=w966, y=w992) -> (x <= y?=w990:bool[])
          n409 = Greater Or Equal?(x=w1018, y=w1019) -> (x >= y?=w1016:bool[])
          n410 = Less Or Equal?(x=w1018, y=w1017) -> (x <= y?=w1015:bool[])
          n411 = Greater Or Equal?(x=w1006, y=w1011) -> (x >= y?=w1009:bool[])
          n412 = Less Or Equal?(x=w1006, y=w1010) -> (x <= y?=w1008:bool[])
          n413 = And(x=w991, y=w990) -> (x .and. y?=→"SHOK?":bool[])
          n414 = Greater Or Equal?(x=w997, y=w1002) -> (x >= y?=w1000:bool[])
          n415 = Less Or Equal?(x=w997, y=w1001) -> (x <= y?=w999:bool[])
          n416 = And(x=w1016, y=w1015) -> (x .and. y?=→"AIs1OK?":bool[])
          n417 = And(x=w1009, y=w1008) -> (x .and. y?=→"AIs2OK?":bool[])
          n418 = And(x=w1000, y=w999) -> (x .and. y?=→"AIs3OK?":bool[])
          n419 = To Long Integer(number=w1034) -> (32bit integer=→"Big Ben, Methodenzeit, Zykluszeit0, Zykluszeit1, Zykluszeit2A, Zykluszeit2B":i32[])
          n420 = Equal?(x=w1047, y=w1046) -> (x = y?=w1045:bool)
          n421 = call "AnzeigeGV_ECD.vi"("veränderte Methode benutzen"=w1084, "Zykluslängen [s]"=w1051, "Cluster1"=w1083, "Big Ben, Methodenzeit, Zykluszeit0, Zykluszeit1, Zykluszeit2A, Zykluszeit2B"=w1034, "Zyklusnummern 0, 1, 2A, 2B"=w1054, "Cluster2"=w1082, "AnzeigeEinstellungen"=w1081, "dargestellte Größe 1"="dargestellte Größe 1", "Zeitachse1"="Zeitachse1", "dargestellte Größe 2"="dargestellte Größe 2", "Zeitachse2"="Zeitachse2") -> ("Anzeige2"=→"Housekeeping2":cluster{dbl[], dbl[]}, "Cluster1"=w1076:cluster{dbl[], dbl[], dbl[], dbl[]}, "x1Inkr"=w1071:dbl, "Cluster2"=w1075:cluster{dbl[], dbl[], dbl[], dbl[]}, "Anzeige1"=→"Housekeeping1":cluster{dbl[], dbl[]}, "AnzeigeEinstellungen"=w1073:T5, "x2Max"=w1035:dbl, "x2Inkr"=w1070:dbl, "x1Max"=w1036:dbl)  [unwired: 8 in]
          n422 = Divide(x=w1049, y=20.0) -> (x/y=w1050:dbl)
          n423 = property on="Detektor 2" class="XYGraph (strikt)"("XScale.Minimum"=w1052, "XScale.Maximum"=w1049, "XScale.Increment"=w1050, "YScale.Minimum"="DetYMin", "YScale.Maximum"="DetYMax", "YScale.Increment"=w1055) -> ()  [unwired: 2 in, 2 out]
          n424 = property on="Housekeeping1" class="XYGraph (strikt)"("XScale.Minimum"=w1052, "XScale.Maximum"=w1036, "XScale.Increment"=w1071, "YScale.Minimum"="HK1YMin", "YScale.Maximum"="HK1YMax", "YScale.Increment"=w1065) -> ()  [unwired: 2 in, 2 out]
          n425 = property on="Housekeeping2" class="XYGraph (strikt)"("XScale.Minimum"=w1052, "XScale.Maximum"=w1035, "XScale.Increment"=w1070, "YScale.Minimum"="HK2YMin", "YScale.Maximum"="HK2YMax", "YScale.Increment"=w1060) -> ()  [unwired: 2 in, 2 out]
          n426 = Select(t=w1043, s=w1045, f=w1044) -> (s? t:f=w1038:cluster{dbl[], dbl[]})
          n427 = Select(t=w1038, s=w1039, f=cluster{dbl[], dbl[]} {[], []} ("s? t:f")) -> (s? t:f=w1031:cluster{dbl[], dbl[]})
          n428 = Build Array(w1042, w1031) -> (→"Detektor 2":cluster{dbl[], "ECD2Chrom":dbl[]}[])
        }
        n429 = while "ZyklusSteuerung" {
          tunnel: w776 -> [w1122]
          tunnel: w777 -> [w1118]
          shift-right: [w1120] -> _
          shift-left: w751 -> [w1126]
          tunnel: w759 -> [w1127]
          tunnel: w677 -> [w1123]
          tunnel: w676 -> [w1124]
          tunnel: w675 -> [w1125]
          shift-right: [w1119] -> _
          shift-left: errorcluster {"status"=FALSE, "code"=0, "source"=""} ("error out") -> [w1121]
          stop <- w1128 stop-if-true
          n430 = call "Bis zum nächsten Vielfachen warten11"("Count(mSec)"=u32 100) -> ()  [unwired: 1 out]
          n431 = global read "GVMethodenwechsel_ECD.vi" "Methodenwechsel?"() -> (w1131:bool)
          n432 = global read "gvbooleschRT_ECD.vi" "global stop RT"() -> (w1130:bool)
          n433 = local read "veränderte Methode benutzen"() -> (w1129:bool)
          n434 = Compound Arithmetic op=OR(w1131, w1130, w1129) -> (w1128:bool)
          n435 = call "ZyklussteuerungGV_ECD.vi"("Traps/MachKoeff0"=w1123, "DIOsNummern"=w1122, "error in"=w1121, "Traps/MachKoeff1"=w1124, "FPGA-VI-Referenz (Ausgang)"=w1118, "Traps/MachKoeff2"=w1125, "Schieberegister"=w1126, "Zeitpunkte/Setpoints"=w1127) -> ("Schieberegister"=w1120:T17, "error out"=w1119:errorcluster)  [unwired: 6 in]
          "Zyklus" <- w1119
        }
        n436 = global read "GVZeitenZyklen_ECD.vi" "Big Ben, Methodenzeit, Zykluszeit0, Zykluszeit1, Zykluszeit2A, Zykluszeit2B"() -> (w738:dbl[])
        n437 = Index Array(array=w738, index=3 ("Index")) -> (element=w736:dbl)
        n438 = while {
          tunnel: w780 -> [w904]
          tunnel: w779 -> [w903]
          tunnel: w702 -> [w918]
          shift-right: [w919] -> w773
          shift-left: w778 -> [w920]
          tunnel: w699 -> [w914]
          tunnel: w698 -> [w908]
          shift-right: [w905] -> _
          shift-left: w736 -> [w909]
          stop <- w921 stop-if-true
          n439 = Less?(x=w909, y=w914) -> (x < y?=w912:bool)
          n440 = Less?(x=w909, y=w908) -> (x < y?=w910:bool)
          n441 = call "Bis zum nächsten Vielfachen warten13"("Count(mSec)"=u32 100 ("Zu wartende ms")) -> ()  [unwired: 1 out]
          n442 = global read "GVMethodenwechsel_ECD.vi" "Methodenwechsel?"() -> (w923:bool)
          n443 = global read "gvbooleschRT_ECD.vi" "global stop RT"() -> (w924:bool)
          n444 = local read "veränderte Methode benutzen"() -> (w922:bool)
          n445 = Compound Arithmetic op=OR(w924, w923, w922) -> (w921:bool)
          n446 = global read "GVZeitenZyklen_ECD.vi" "Big Ben, Methodenzeit, Zykluszeit0, Zykluszeit1, Zykluszeit2A, Zykluszeit2B"() -> (w916:dbl[])
          n447 = Index Array(array=w916, index=3 ("Index")) -> (element=w905:dbl)
          n448 = Greater Or Equal?(x=w905, y=w914) -> (x >= y?=w913:bool)
          n449 = Greater Or Equal?(x=w905, y=w908) -> (x >= y?=w911:bool)
          n450 = And(x=w911, y=w910) -> (x .and. y?=w907:bool)
          n451 = And(x=w913, y=w912) -> (x .and. y?=w902:bool)
          n452 = Or(x=w902, y=w907) -> (x .or. y?=w906:bool)
          n453 = And(x=w918, y=w906) -> (x .and. y?=w917:bool)
          n454 = case shown="True" w917 {
            tunnel: w920 -> [w926 w927]
            tunnel: [w926 w931] -> w919
            tunnel: w904 -> [_ w930]
            tunnel: w903 -> [_ w929]
            tunnel: w902 -> [_ w928]
            frame False {
            }
            frame True {
              n455 = call "MSDateienSchicken_ECD.vi"("MSNummer"=w927, "MSa?"=w928, "Dateipfad:fromcriordy"=w929, "Dateipfad:fromcriocmd"=w930) -> ()  [unwired: 1 in]
              n456 = Increment(x=w927) -> (x+1=w931:i32)
            }
          }
        }
      }
      n457 = case shown="True" TRUE ("HKSpeichern") {
        tunnel: w418 -> [_ w647]
        frame False {
        }
        frame True {
          n458 = while {
            tunnel: w647 -> [w651]
            shift-right: [w649] -> _
            shift-left: errorcluster {"status"=FALSE, "code"=0, "source"=""} ("error out") -> [w648]
            stop <- w653 stop-if-true
            n459 = call "Bis zum nächsten Vielfachen warten2"("Count(mSec)"=u32 1000) -> ()  [unwired: 1 out]
            n460 = local read "Methode"() -> (w650:i32)
            n461 = global read "gvbooleschRT_ECD.vi" "global stop RT"() -> (w653:bool)
            n462 = call "HKinTDMS_ECD.vi"("Methode"=w650, "error in (no error)"=w648, "Kanäle"=w651) -> ("error out"=w649:errorcluster)
            "TDMSwriteHK" <- w649
          }
        }
      }
      n463 = Concatenate Strings("?SE0,GDATA" ("Schreibpuffer"), "\r") -> (w324:string)
      n464 = Build Array(w383, w382, w381) -> (w380:i32[])
      n465 = Add Array Elements(numeric array=w380) -> (sum=w390:i32)
      n466 = Index Array(array=w380, index #1=0 ("Index"), index #2=1 ("Index")) -> (element #1=w401:i32, element #2=w399:i32)
      n467 = while {
        stop <- w1193 stop-if-true
        w1187 = 10.0
        n468 = call "Warten2"("Count(mSec)"=u32 1000) -> ()  [unwired: 1 out]
        n469 = global read "gvbooleschRT_ECD.vi" "global stop RT"() -> (w1193:bool)
        n470 = global read "GVTrapsMachs_ECD.vi" "Traps/Machs"() -> (w1183:dbl[])
        n471 = global read "GVAIs_ECD.vi" "AIs"() -> (w1184:dbl[])
        n472 = for {
          N: 9 -> [_]
          shift-right: [w1196] -> w1190
          shift-left: w1184 -> [w1197]
          shift-right: [w1194] -> w1188
          shift-left: w1183 -> [w1195]
          n473 = flat-sequence {
            tunnel: w1197 -> [w1204]
            tunnel: [w1203] -> w1196
            tunnel: w1195 -> [w1202]
            tunnel: [w1201] -> w1194
            frame #0 {
              n474 = call "Warten28"("Count(mSec)"=u32 100) -> ()  [unwired: 1 out]
            }
            frame #1 {
              n475 = global read "GVAIs_ECD.vi" "AIs"() -> (w1200:dbl[])
              n476 = Add(x=w1204, y=w1200) -> (x+y=w1203:dbl[])
              n477 = global read "GVTrapsMachs_ECD.vi" "Traps/Machs"() -> (w1199:dbl[])
              n478 = Add(x=w1199, y=w1202) -> (x+y=w1201:dbl[])
            }
          }
        }
        n479 = Divide(x=w1190, y=w1187) -> (x/y=w1189:dbl[])
        n480 = Divide(x=w1188, y=w1187) -> (x/y=w1186:dbl[])
        n481 = Build Array (concatenate)(w1189, w1186) -> (w1185:dbl[])
        n482 = global write "GVHK1Hz_ECD.vi" "Mod1Mod2Mod3/AITrapsMachs1Hz"(w1185) -> ()
      }
      n483 = Split 1D Array(array=w379, index=w401) -> (first subarray=w405:dbl[], second subarray=w409:dbl[])
      n484 = Split 1D Array(array=w377, index=w401) -> (first subarray=w408:string[], second subarray=w410:string[])
      n485 = Split 1D Array(array=w378, index=w401) -> (first subarray=w398:string[], second subarray=w400:string[])
      n486 = Initialize Array(-1.0 ("Element"), w390) -> (w375:dbl[])
      n487 = case shown="True" TRUE ("ECDSpeichern") {
        frame False {
        }
        frame True {
          w594 = dbl[] []
          n488 = global read "GVaktuelleTDMS_ECD.vi" "aktuelleTDMS-DateiECD1"() -> (w595:refnum<k34>)
          n489 = while {
            shift-right: [w607] -> _
            shift-left: w594 -> [w611]
            shift-right: [w600] -> _
            shift-left: w594 -> [w604]
            shift-right: [w606] -> _
            shift-left: w595 -> [w609]
            tunnel: w594 -> [w603]
            shift-right: [w597] -> _
            shift-left: errorcluster {"status"=FALSE, "code"=0, "source"=""} ("error IO") -> [w596]
            stop <- w616 stop-if-true
            n490 = call "Bis zum nächsten Vielfachen warten3"("Count(mSec)"=u32 500) -> ()  [unwired: 1 out]
            n491 = global read "GVECDs_ECD.vi" "ECD1MW"() -> (w610:dbl[])
            n492 = global read "GVECDs_ECD.vi" "ECD2MW"() -> (w601:dbl[])
            n493 = global read "gvbooleschRT_ECD.vi" "global stop RT"() -> (w616:bool)
            n494 = Build Array (concatenate)(w611, w610) -> (w608:dbl[])
            n495 = Build Array (concatenate)(w604, w601) -> (w605:dbl[])
            n496 = global read "GVaktuelleTDMS_ECD.vi" "aktuelleTDMS-DateiECD1"() -> (w606:refnum<k34>)
            n497 = global read "GVaktuelleTDMS_ECD.vi" "aktuelleTDMS-DateiECD2"() -> (w614:refnum<k34>)
            n498 = Equal?(x=w609, y=w606) -> (x = y?=w602:bool)
            n499 = TDMS Write(0:w606, 7:"ECD1", 9:w610, 11:w596) -> (15:w599:errorcluster)  [unwired: 2 in, 3 out]
            n500 = TDMS Write(0:w614, 7:"ECD2", 9:w601, 11:w596) -> (15:w598:errorcluster)  [unwired: 2 in, 3 out]
            n501 = Select(t=w608, s=w602, f=w603) -> (s? t:f=w607:dbl[])
            n502 = Select(t=w605, s=w602, f=w603) -> (s? t:f=w600:dbl[])
            n503 = global write "GVChroms_ECD.vi" "ECD1Chrom"(w607) -> ()
            n504 = global write "GVChroms_ECD.vi" "ECD2Chrom"(w600) -> ()
            n505 = Merge Errors(w599, w598) -> (w597:errorcluster)
            "TDMSwriteECD" <- w597
          }
        }
      }
      n506 = while {
        shift-right: [w423] -> _
        shift-left: w323 -> [w425]
        shift-right: [w422] -> _
        shift-left: w323 -> [w424]
        stop <- w427 stop-if-true
        n507 = call "Bis zum nächsten Vielfachen warten"("Count(mSec)"=u32 100) -> ()  [unwired: 1 out]
        n508 = case shown="True" "An/Aus" {
          tunnel: w425 -> [w429 w445]
          tunnel: w424 -> [w428 w444]
          tunnel: [w429 w438] -> w423
          tunnel: [w428 w437] -> w422
          frame False {
          }
          frame True {
            w441 = dbl[] [] ("t")
            n509 = global read "GVMWHorst_ECD.vi" "MWHorst"() -> (w434:dbl[])
            n510 = global read "GVTrapsMachs_ECD.vi" "Traps/Machs"() -> (w435:dbl[])
            n511 = Build Array (concatenate)(w435, w434) -> (w433:dbl[])
            n512 = Index Array(array=w433, index="dargestellte Größe 3") -> (element=w446:dbl)
            n513 = Build Array (concatenate)(w445, w446) -> (w439:dbl[])
            n514 = Select(t=w441, s="TafelWischen!", f=w439) -> (s? t:f=w438:dbl[])
            n515 = global read "GVZeitenZyklen_ECD.vi" "Big Ben, Methodenzeit, Zykluszeit0, Zykluszeit1, Zykluszeit2A, Zykluszeit2B"() -> (w432:dbl[])
            n516 = Index Array(array=w432, index=1 ("Index")) -> (element=w430:dbl)
            n517 = Build Array (concatenate)(w444, w430) -> (w440:dbl[])
            n518 = Select(t=w441, s="TafelWischen!", f=w440) -> (s? t:f=w437:dbl[])
            n519 = Bundle(w440, w439) -> (→"schnelleAnzeige":cluster{dbl[], dbl[]})  [unwired: 1 in]
          }
        }
        n520 = global read "gvbooleschRT_ECD.vi" "global stop RT"() -> (w427:bool)
      }
      n521 = case shown="True" TRUE {
        tunnel: w369 -> [_ w626]
        tunnel: w367 -> [_ w625]
        tunnel: w366 -> [_ w624]
        tunnel: w361 -> [_ w623]
        tunnel: w360 -> [_ w622]
        frame False {
        }
        frame True {
          w617 = errorcluster {"status"=FALSE, "code"=0, "source"=""} ("error out TDMSopen")
          n522 = while {
            shift-right: [w631] -> w621
            shift-left: w623 -> [w633]
            shift-right: [w642] -> w620
            shift-left: w622 -> [w635]
            shift-right: [w637] -> _
            shift-left: w626 -> [w643]
            tunnel: w624 -> [w639]
            tunnel: w625 -> [w640]
            shift-right: [w630] -> w619
            shift-left: w617 -> [w628]
            shift-right: [w629] -> w618
            shift-left: w617 -> [w627]
            stop <- w645 stop-if-true
            n523 = call "Bis zum nächsten Vielfachen warten5"("Count(mSec)"=u32 500) -> ()  [unwired: 1 out]
            n524 = local read "Methode"() -> (w641:i32)
            n525 = global read "gvbooleschRT_ECD.vi" "global stop RT"() -> (w645:bool)
            n526 = global read "GVZeitenZyklen_ECD.vi" "ZyklusNummernGesamt"() -> (w632:i32[])
            n527 = Index Array(array=w632, index=1 ("Index")) -> (element=w637:i32)
            n528 = Greater?(x=w637, y=w643) -> (0:w636:bool)
            n529 = Select(t=w635, s=w636, f=w633) -> (s? t:f=w634:refnum<k34>)
            n530 = call "AktuelleTDMS_ECD.vi"("AktuelleTDMS"=w633, "error in TDMSopen"=w628, "Dateiordner"=w640, "NächsteTDMS"=w635, "NeuerZyklus?"=w636, "Methodennummer"=w641, "Zyklnumges"=w637, "error in TDMSclose"=w627, "Dateiname"=w639) -> ("AktuelleTDMS"=w631:refnum<k34>, "error out TDMSopen"=w630:errorcluster, "error out TDMSclose"=w629:errorcluster, "NächsteTDMS"=w642:refnum<k34>)  [unwired: 3 in]
            "TDMSopenHK" <- w630
            "TDMScloseHK" <- w629
            n531 = global write "GVaktuelleTDMS_ECD.vi" "aktuelleTDMS-DateiHK"(w634) -> ()
          }
          n532 = TDMS Close(8:w619, 11:w621) -> ()  [unwired: 2 out]
          n533 = TDMS Close(8:w618, 11:w620) -> ()  [unwired: 2 out]
        }
      }
      n534 = case shown="True" TRUE {
        tunnel: w369 -> [_ w554]
        tunnel: w365 -> [_ w553]
        tunnel: w364 -> [_ w552]
        tunnel: w363 -> [_ w551]
        tunnel: w362 -> [_ w550]
        tunnel: w359 -> [_ w549]
        tunnel: w358 -> [_ w548]
        tunnel: w357 -> [_ w547]
        tunnel: w356 -> [_ w546]
        frame False {
        }
        frame True {
          w539 = errorcluster {"status"=FALSE, "code"=0, "source"=""} ("error out TDMSopen")
          n535 = while {
            shift-right: [w578] -> w545
            shift-left: w549 -> [w580]
            shift-right: [w588] -> w544
            shift-left: w548 -> [w582]
            shift-right: [w586] -> _
            shift-left: w554 -> [w589]
            tunnel: w553 -> [w585]
            tunnel: w551 -> [w584]
            shift-right: [w577] -> w540
            shift-left: w539 -> [w575]
            shift-right: [w576] -> w541
            shift-left: w539 -> [w574]
            stop <- w591 stop-if-true
            n536 = call "Bis zum nächsten Vielfachen warten4"("Count(mSec)"=u32 500) -> ()  [unwired: 1 out]
            n537 = local read "Methode"() -> (w587:i32)
            n538 = global read "gvbooleschRT_ECD.vi" "global stop RT"() -> (w591:bool)
            n539 = global read "GVZeitenZyklen_ECD.vi" "ZyklusNummernGesamt"() -> (w579:i32[])
            n540 = Index Array(array=w579, index=2 ("Index")) -> (element=w586:i32)
            n541 = Greater?(x=w586, y=w589) -> (0:w583:bool)
            n542 = Select(t=w582, s=w583, f=w580) -> (s? t:f=w581:refnum<k34>)
            n543 = call "AktuelleTDMS_ECD.vi"("AktuelleTDMS"=w580, "error in TDMSopen"=w575, "Dateiordner"=w585, "NächsteTDMS"=w582, "NeuerZyklus?"=w583, "Methodennummer"=w587, "Zyklnumges"=w586, "error in TDMSclose"=w574, "Dateiname"=w584) -> ("AktuelleTDMS"=w578:refnum<k34>, "error out TDMSopen"=w577:errorcluster, "error out TDMSclose"=w576:errorcluster, "NächsteTDMS"=w588:refnum<k34>)  [unwired: 3 in]
            "TDMSopenECD1" <- w577
            "TDMScloseECD1" <- w576
            n544 = global write "GVaktuelleTDMS_ECD.vi" "aktuelleTDMS-DateiECD1"(w581) -> ()
          }
          n545 = while {
            shift-right: [w568] -> w543
            shift-left: w547 -> [w560]
            shift-right: [w569] -> w542
            shift-left: w546 -> [w562]
            shift-right: [w566] -> _
            shift-left: w554 -> [w570]
            tunnel: w552 -> [w565]
            tunnel: w550 -> [w564]
            shift-right: [w558] -> _
            shift-left: w539 -> [w556]
            shift-right: [w557] -> _
            shift-left: w539 -> [w555]
            stop <- w572 stop-if-true
            n546 = call "Bis zum nächsten Vielfachen warten6"("Count(mSec)"=u32 500) -> ()  [unwired: 1 out]
            n547 = local read "Methode"() -> (w567:i32)
            n548 = global read "gvbooleschRT_ECD.vi" "global stop RT"() -> (w572:bool)
            n549 = global read "GVZeitenZyklen_ECD.vi" "ZyklusNummernGesamt"() -> (w559:i32[])
            n550 = Index Array(array=w559, index=3 ("Index")) -> (element=w566:i32)
            n551 = Greater?(x=w566, y=w570) -> (0:w563:bool)
            n552 = Select(t=w562, s=w563, f=w560) -> (s? t:f=w561:refnum<k34>)
            n553 = call "AktuelleTDMS_ECD.vi"("AktuelleTDMS"=w560, "error in TDMSopen"=w556, "Dateiordner"=w565, "NächsteTDMS"=w562, "NeuerZyklus?"=w563, "Methodennummer"=w567, "Zyklnumges"=w566, "error in TDMSclose"=w555, "Dateiname"=w564) -> ("AktuelleTDMS"=w568:refnum<k34>, "error out TDMSopen"=w558:errorcluster, "error out TDMSclose"=w557:errorcluster, "NächsteTDMS"=w569:refnum<k34>)  [unwired: 3 in]
            "TDMSopenECD2" <- w558
            "TDMScloseECD2" <- w557
            n554 = global write "GVaktuelleTDMS_ECD.vi" "aktuelleTDMS-DateiECD2"(w561) -> ()
          }
          n555 = TDMS Close(8:w540, 11:w545) -> ()  [unwired: 2 out]
          n556 = TDMS Close(8:w541, 11:w544) -> ()  [unwired: 2 out]
          n557 = TDMS Close(11:w543) -> ()  [unwired: 1 in, 2 out]
          n558 = TDMS Close(11:w542) -> ()  [unwired: 1 in, 2 out]
        }
      }
      n559 = Split 1D Array(array=w410, index=w399) -> (first subarray=w407:string[], second subarray=w406:string[])
      n560 = Split 1D Array(array=w409, index=w399) -> (first subarray=w404:dbl[], second subarray=w403:dbl[])
      n561 = Split 1D Array(array=w400, index=w399) -> (first subarray=w397:string[], second subarray=w396:string[])
      n562 = Bundle(w408, w407, w406, w405, w404, w403) -> (w402:T18)  [unwired: 1 in]
      n563 = Bundle(w398, w397, w396) -> (w395:cluster{string[], string[], string[]})  [unwired: 1 in]
      n564 = Initialize Array(0.0, 8 ("Dimension")) -> (w325:dbl[])
      n565 = Bundle(w394, w394, w394) -> (w393:cluster{i32, i32, i32})  [unwired: 1 in]
      n566 = Initialize Array("x", 8 ("Dimension")) -> (w330:string[])
      n567 = case shown="True" TRUE ("SerielleKomm.") {
        tunnel: bool[] [TRUE, TRUE, TRUE, TRUE, TRUE, TRUE, TRUE, TRUE] -> [_ w463]
        tunnel: w330 -> [_ w462]
        tunnel: w402 -> [_ w461]
        tunnel: w401 -> [_ w460]
        tunnel: w399 -> [_ w459]
        tunnel: w395 -> [_ w458]
        tunnel: w393 -> [_ w457]
        tunnel: w392 -> [_ w456]
        tunnel: w379 -> [_ w455]
        tunnel: w376 -> [_ w454]
        tunnel: w375 -> [_ w453]
        tunnel: w374 -> [_ w450]
        tunnel: w353 -> [_ w452]
        tunnel: w325 -> [_ w451]
        tunnel: w324 -> [_ w449]
        frame False {
        }
        frame True {
          n568 = while {
            tunnel: w450 -> [w477]
            tunnel: w449 -> [w476]
            shift-right: [w475] -> _
            shift-left: errorcluster {"status"=FALSE, "code"=0, "source"=""} ("error out") -> [w474]
            stop <- w478 stop-if-true
            n569 = call "Warten6"("Count(mSec)"=u32 500) -> ()  [unwired: 1 out]
            n570 = global read "gvbooleschRT_ECD.vi" "global stop RT"() -> (w478:bool)
            n571 = case shown="True" "NeuerRefstrom" {
              tunnel: w476 -> [w480 _]
              tunnel: [w479 w489] -> w469
              tunnel: [w479 w492] -> w465
              frame False {
                n572 = String To Byte Array(string=w480) -> (unsigned byte array=w479:u8[])
              }
              frame True {
                n573 = local write "NeuerRefstrom"(FALSE ("NeuerRefstrom")) -> ()
                n574 = Number To Decimal String(number="RefStromECD1", width (-)=i16 4) -> (decimal integer string=w484:string)
                n575 = Number To Decimal String(number="RefStromECD2", width (-)=i16 4) -> (decimal integer string=w481:string)
                n576 = Concatenate Strings("?SE0,SETP," ("string"), w484, "\n") -> (w493:string)
                n577 = Concatenate Strings("?SE0,SETP," ("string"), w481, "\n") -> (w490:string)
                n578 = String To Byte Array(string=w493) -> (unsigned byte array=w492:u8[])
                n579 = String To Byte Array(string=w490) -> (unsigned byte array=w489:u8[])
              }
            }
            n580 = Join Numbers(hi=w465, lo=u8 5) -> ((hi.lo)=w471:u16[])
            n581 = Join Numbers(hi=w469, lo=u8 6) -> ((hi.lo)=w467:u16[])
            n582 = xnode "Invoke Method"("FPGA-VI-Referenz (Eingang)"=w477, "Fehler (Eingang)"=w474, "Daten"=w471) -> ("FPGA-VI-Referenz (Ausgang)"=w470:refnum<k20>, "Fehler (Ausgang)"=w466:errorcluster)  [unwired: 1 in, 1 out]
            n583 = xnode "Invoke Method"("FPGA-VI-Referenz (Eingang)"=w470, "Fehler (Eingang)"=w466, "Daten"=w467) -> ("Fehler (Ausgang)"=w475:errorcluster)  [unwired: 1 in, 2 out]
            "FIFOwriteRS485" <- w475
          }
          n584 = while {
            shift-right: [w497] -> _
            shift-left: w463 -> [w516]
            shift-right: [w520] -> _
            shift-left: w453 -> [w526]
            tunnel: w450 -> [w513]
            shift-right: [w498] -> _
            shift-left: w462 -> [w496]
            tunnel: w454 -> [w504]
            tunnel: w455 -> [w500]
            shift-right: [w505] -> _
            shift-left: w456 -> [w522]
            tunnel: w460 -> [w524]
            tunnel: w459 -> [w525]
            tunnel: w461 -> [w527]
            tunnel: w458 -> [w510]
            shift-right: [w506] -> _
            shift-left: w457 -> [w509]
            shift-right: [w512] -> _
            shift-left: w452 -> [w515]
            shift-right: [w517] -> _
            shift-left: w451 -> [w518]
            shift-right: [w499] -> _
            shift-left: errorcluster {"status"=FALSE, "code"=0, "source"=""} ("error out") -> [w514]
            stop <- w521 stop-if-true
            n585 = for {
              tunnel: w516 -> [w531] mode=indexing
              tunnel: w518 -> [w528] mode=indexing
              tunnel: [w535] -> w517 mode=indexing
              tunnel: [w532] -> w508 mode=indexing
              n586 = global read "GVZeitenZyklen_ECD.vi" "Big Ben, Methodenzeit, Zykluszeit0, Zykluszeit1, Zykluszeit2A, Zykluszeit2B"() -> (w538:dbl[])
              n587 = Index Array(array=w538, index=0 ("Index")) -> (element=w536:dbl)
              n588 = Subtract(x=w536, y=w528) -> (x-y=w534:dbl)
              n589 = Greater?(x=w534, y=1.0) -> (0:w530:bool)
              n590 = Or(x=w531, y=w530) -> (x .or. y?=w529:bool)
              n591 = Select(t=w530, s=w530, f=w531) -> (s? t:f=w532:bool)
              n592 = Select(t=w536, s=w529, f=w528) -> (s? t:f=w535:dbl)
            }
            n593 = global read "GVHorstSP_ECD.vi" "HorstSP"() -> (w520:dbl[])
            n594 = Not Equal?(x=w520, y=w526) -> (x != y?=w523:bool)
            n595 = call "NeueSP_ECD.vi"("Anzahl2"=w525, "Anzahl1"=w524, "AlteSP"=w526, 7:"NeueSP"=w520, "BefehleCluster"=w522, 10:"NeueSP"=w523, "ClusterFest"=w527) -> ("BefehleCluster"=w507:T19)  [unwired: 4 in]
            n596 = call "Warten3"("Count(mSec)"=u32 100) -> ()  [unwired: 1 out]
            n597 = call "MPVSenden_ECD.vi"("Ventilposition"=w515, "error in"=w514, "FPGA-VI-Referenz (Ausgang) 2"=w513) -> ("Ventilposition"=w512:i32, "error out"=w511:errorcluster, "FPGA-VI-Referenz (Ausgang)"=w503:refnum<k20>)
            n598 = call "Senden_ECD.vi"("error in"=w511, "BefehlsCluster"=w507, "AbfragenCluster"=w510, "Abfragenr.Cluster"=w509, "Senden?"=w508, "FPGA-VI-Referenz (Ausgang)"=w503) -> ("BefehlsCluster"=w505:T19, "error out"=w501:errorcluster, "Senden?"=w502:bool[], "Abfragenr.Cluster"=w506:cluster{i32, i32, i32})  [unwired: 1 in]
            n599 = call "SeriellRead_ECD.vi"("SkalierungsfaktorHorst"=w500, "VorwortHorst"=w504, "error in"=w501, "Zwischenspeicher"=w496, "Senden?"=w502, "FPGA-VI-Referenz (Ausgang)"=w503) -> ("Senden?"=w497:bool[], "Zwischenspeicher"=w498:string[], "error out"=w499:errorcluster)  [unwired: 3 in]
            "SerielleKomm." <- w499
            n600 = global read "gvbooleschRT_ECD.vi" "global stop RT"() -> (w521:bool)
          }
        }
      }
    }
    frame #2 {
      n601 = xnode "Element lesen/schreiben"("FPGA-VI-Referenz (Eingang)"=w1212, "global stop"=TRUE) -> ("FPGA-VI-Referenz (Ausgang)"=w1211:refnum<k20>)  [unwired: 1 in, 1 out]
      n602 = xnode "Close FPGA VI Reference"("FPGA-VI-Referenz (Eingang)"=w1211) -> ()  [unwired: 1 in, 1 out]
    }
    frame #3 {
    }
    frame #4 {
    }
  }
